vi "Master_IMUMain.vi"(8 "error in":errorcluster, 11 "VISA Refnum out":refnum<visa-resource-name>) -> (0 "error out":errorcluster)   [LabVIEW 2018]
doc: "VI dedicated to reading and processing incoming data from IMU (SBG Ellipse)."
panel:
  out "Data skipped":bool
  out "buffer length":i32
  out "msg_id":string
  # "."
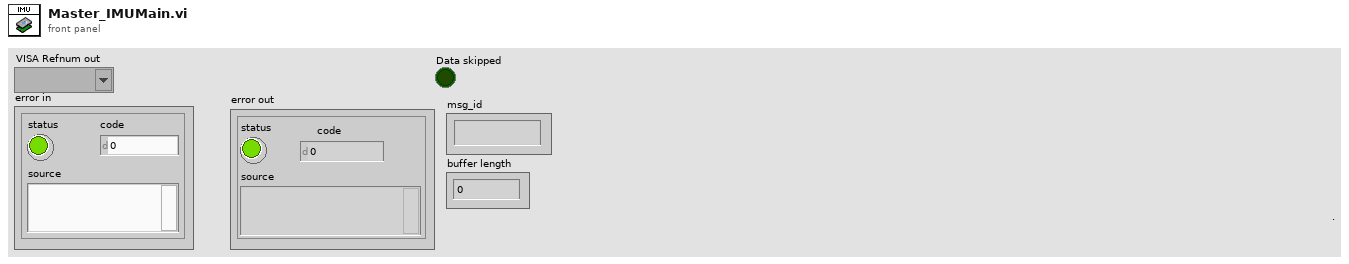
[diagram p1: front panel]
types:
  T1 = cluster{"x acceleration (g)":dbl, "Pressure (psia)":dbl, "Temperature (F)":dbl}
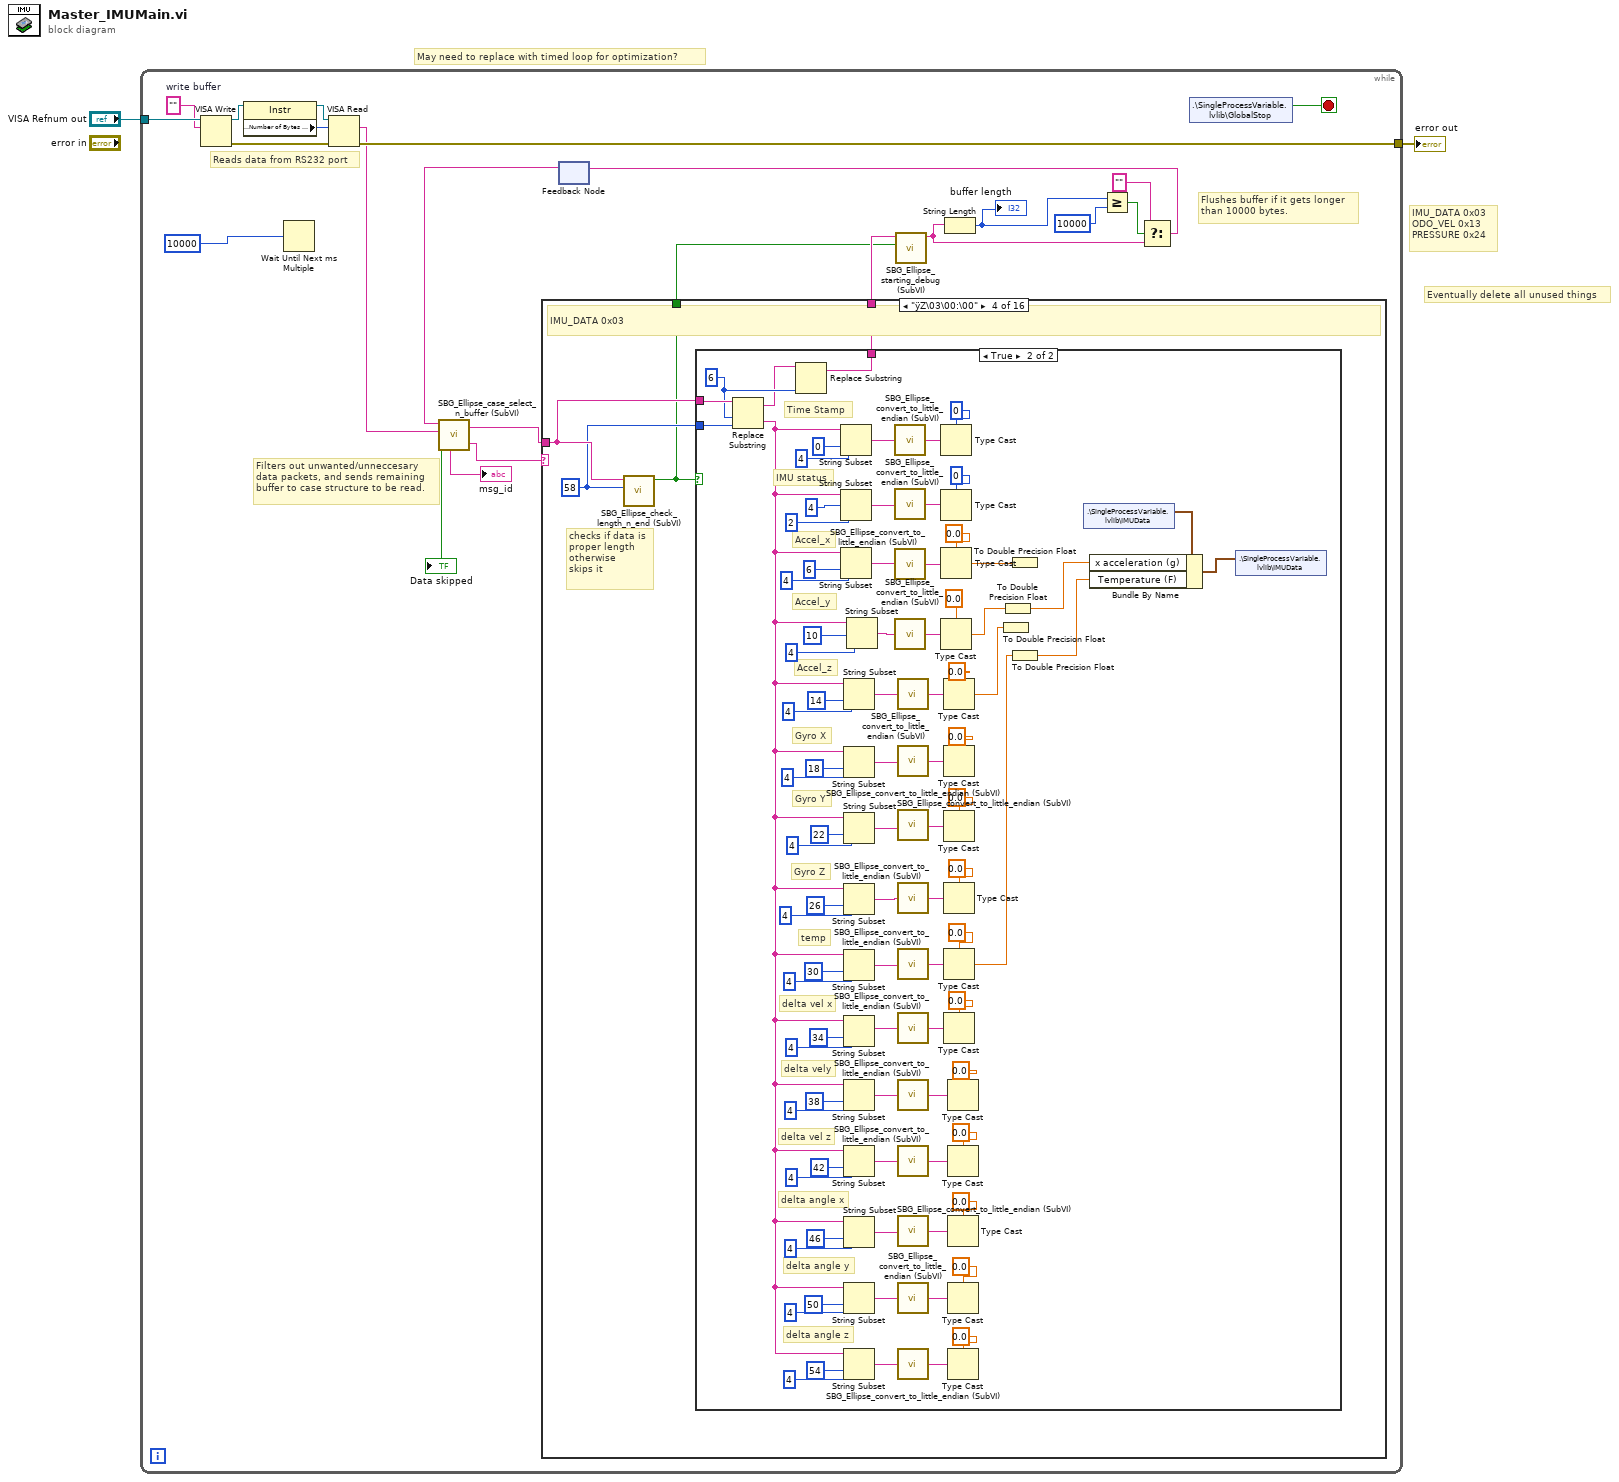
[diagram p0: block diagram]
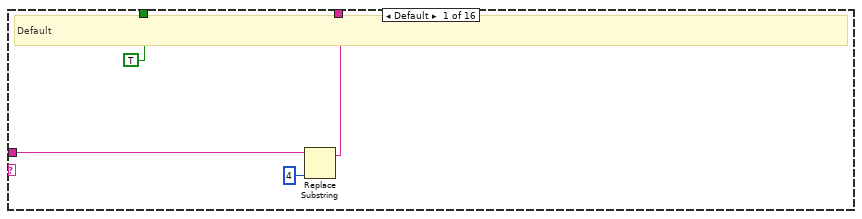
[diagram p2: hidden frame]
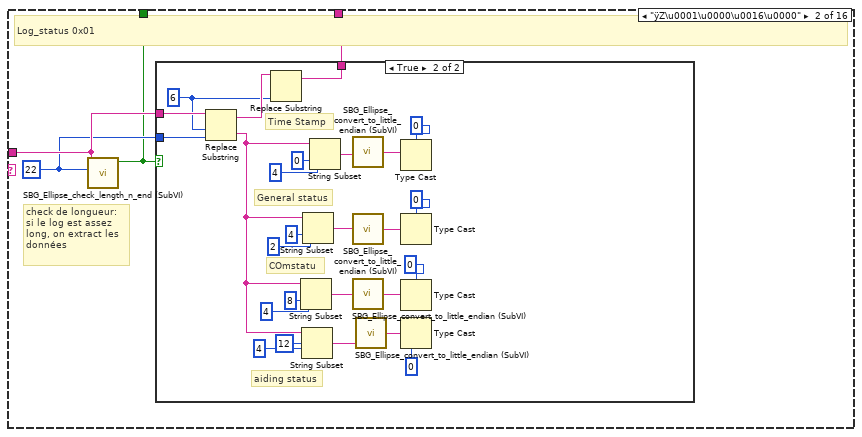
[diagram p3: hidden frame]
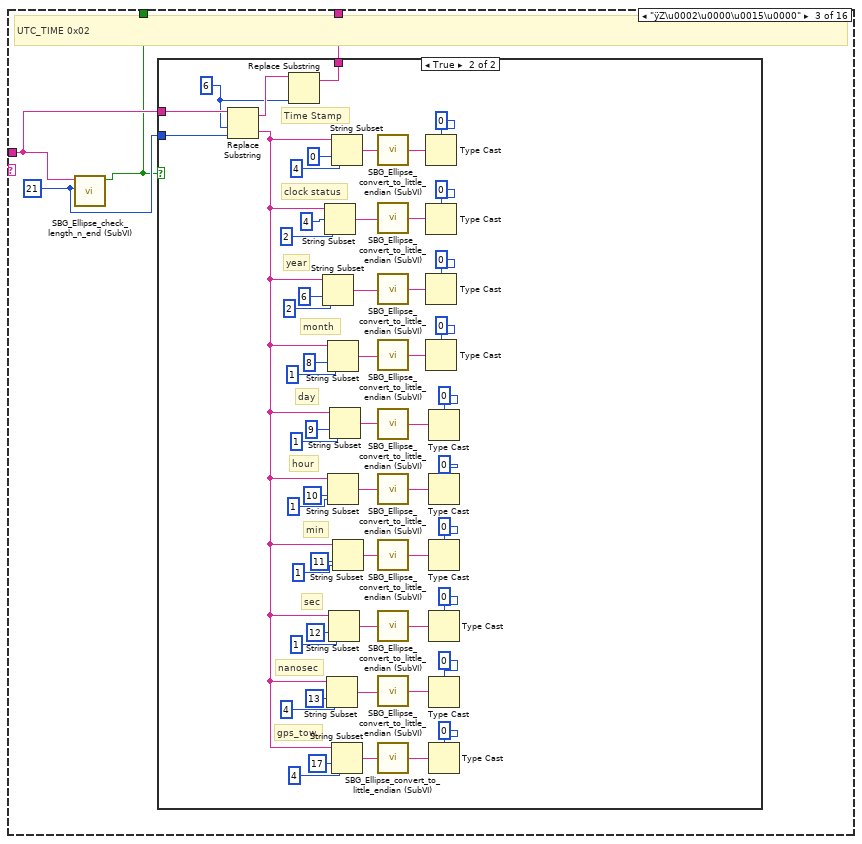
[diagram p5: hidden frame]
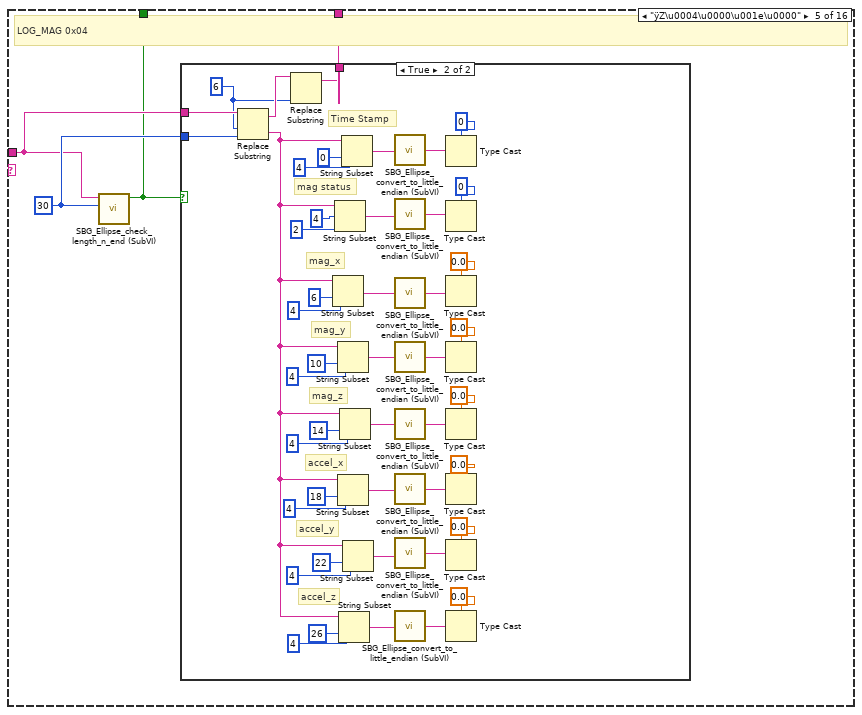
[diagram p8: hidden frame]
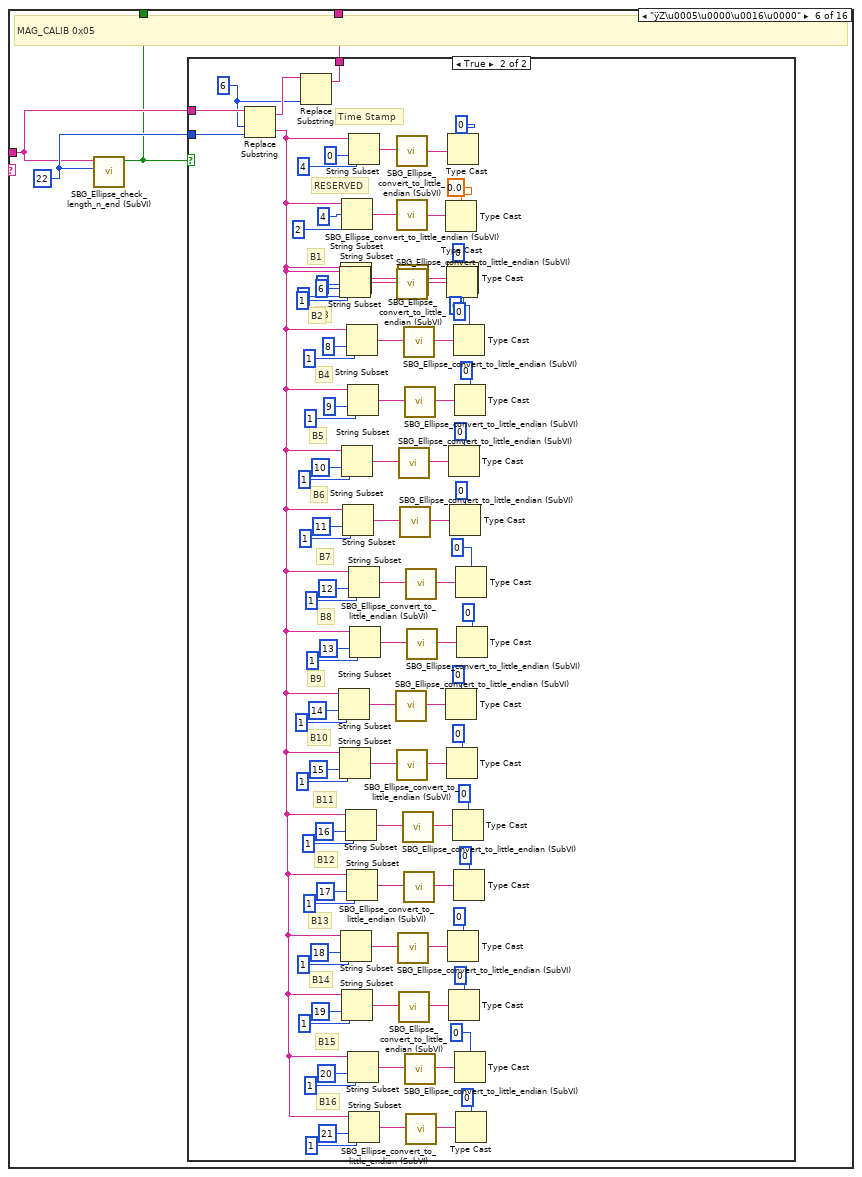
[diagram p10: hidden frame]
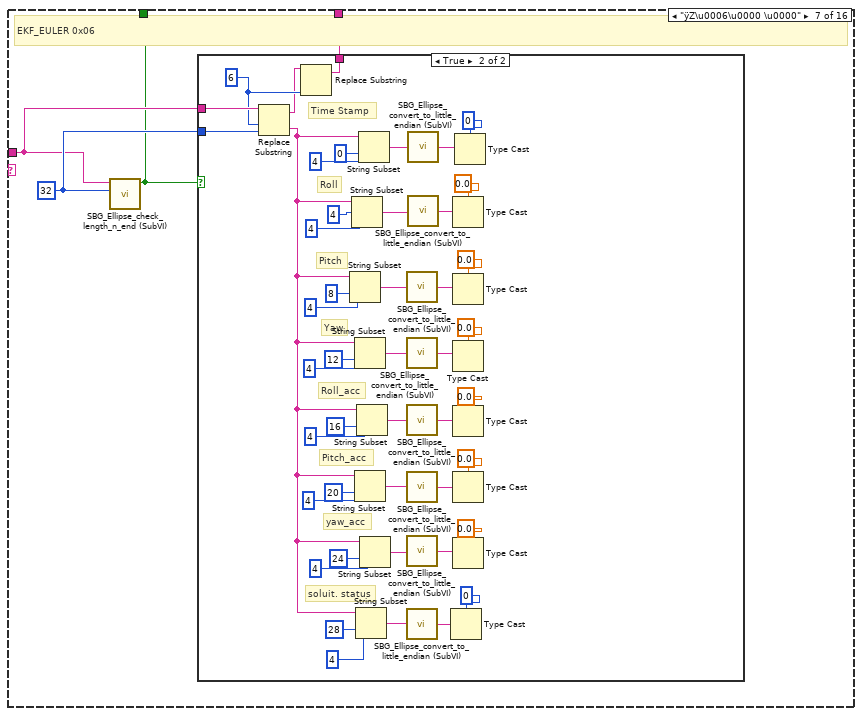
[diagram p12: hidden frame]
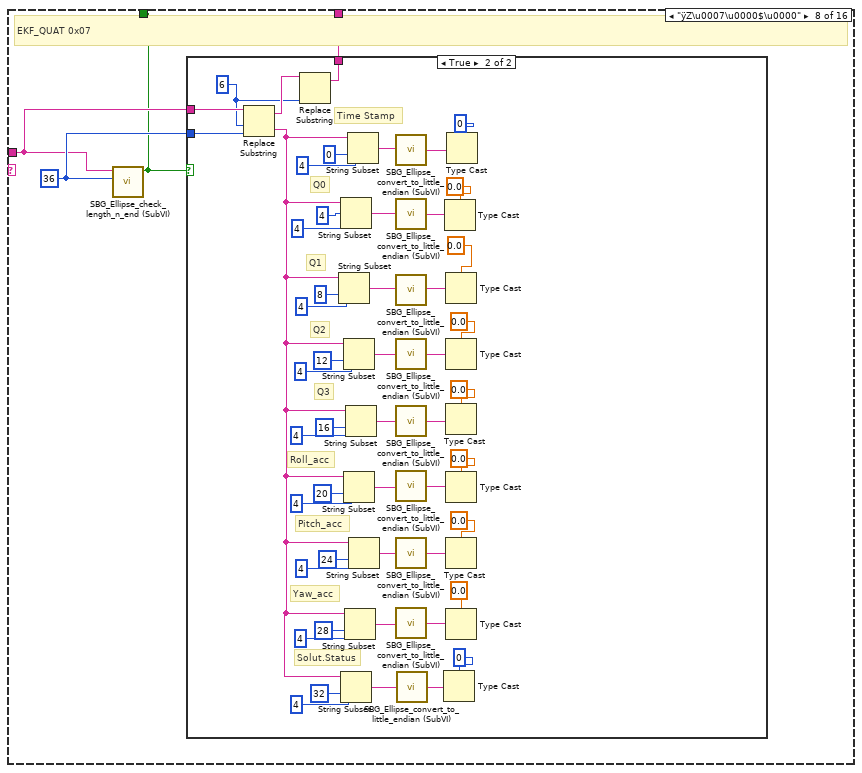
[diagram p14: hidden frame]
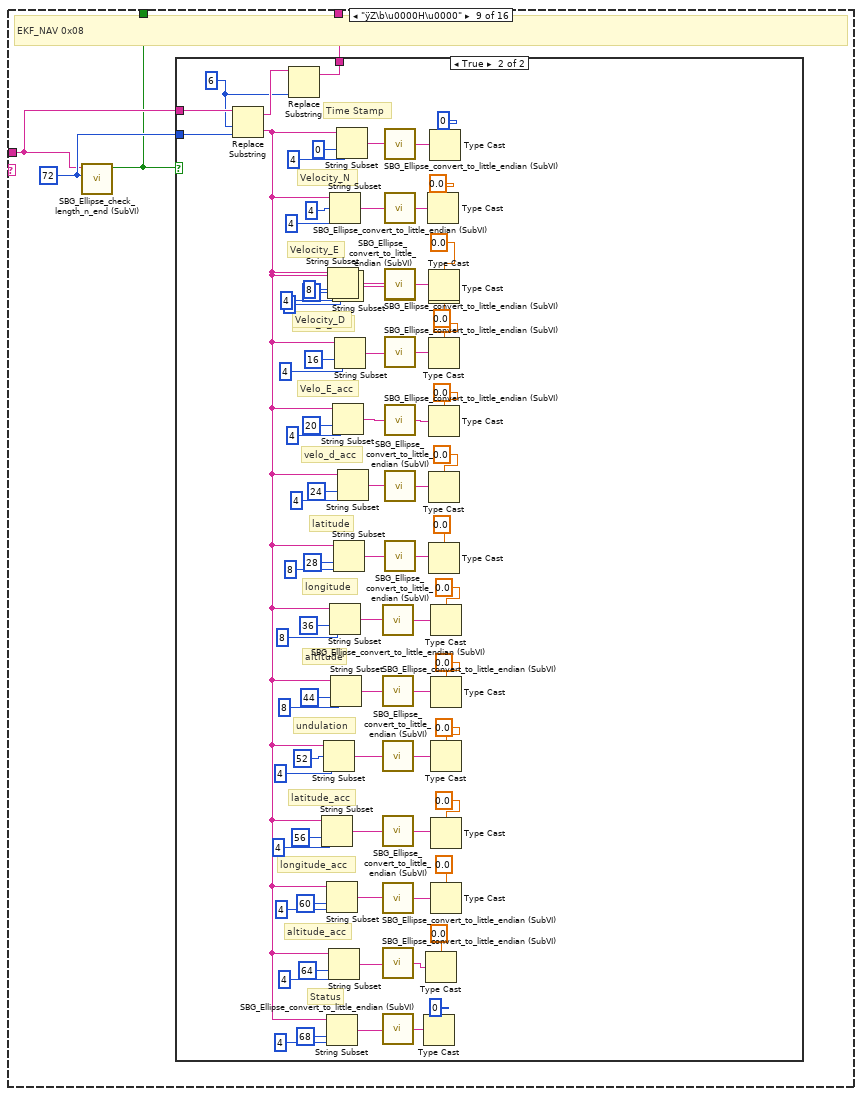
[diagram p16: hidden frame]
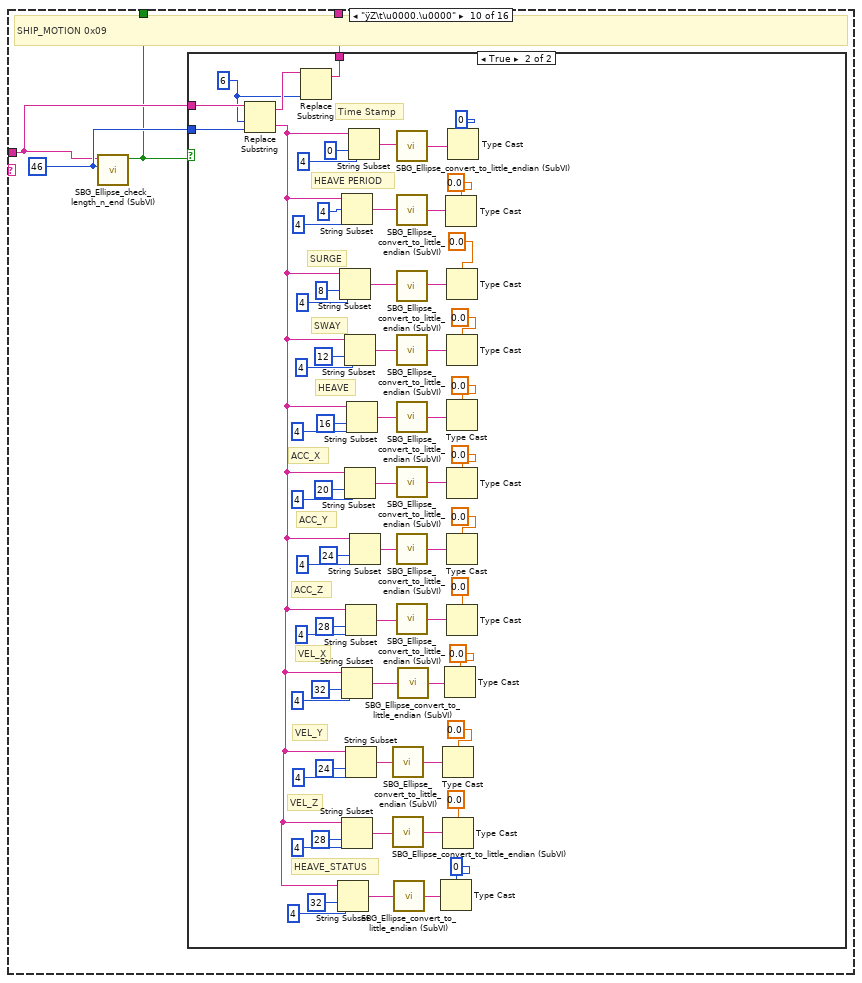
[diagram p18: hidden frame]
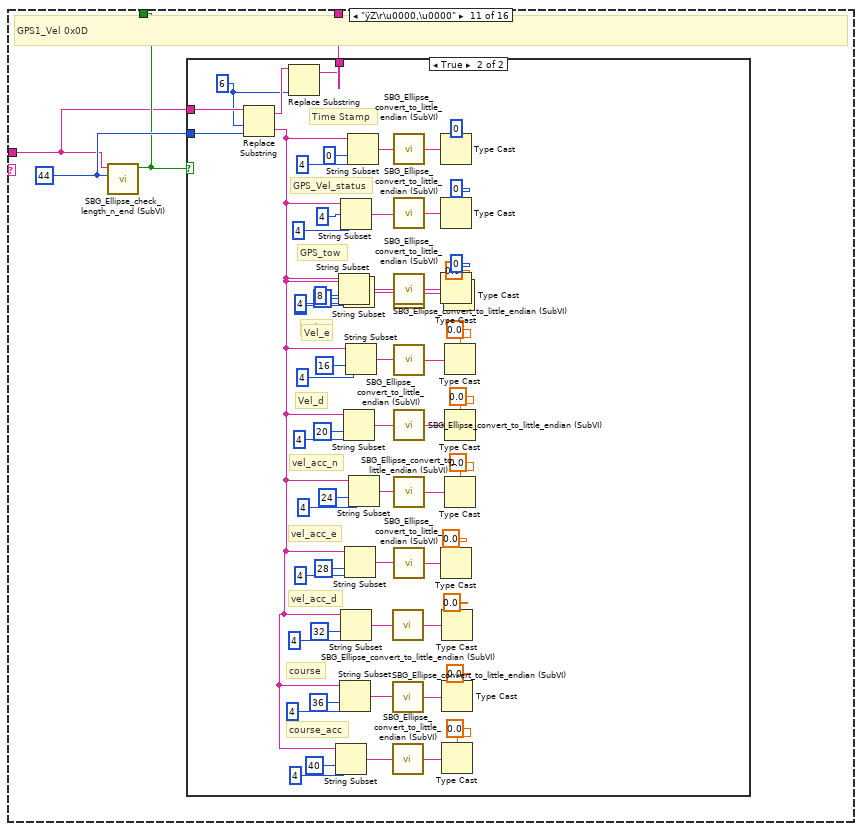
[diagram p20: hidden frame]
diagram:
  # "Eventually delete all unused things"
  # "May need to replace with timed loop for optimization?"
  # "IMU_DATA 0x03\nODO_VEL 0x13\nPRESSURE 0x24"
  n1 = while {
    tunnel: "VISA Refnum out" -> [w25]
    tunnel: [w19] -> w1
    stop <- w9 stop-if-true
    w20 = ""  # write buffer
    # "Filters out unwanted/unneccesary \ndata packets, and sends remaining\nbuffer to case structure to be read."
    # "Reads data from RS232 port"
    # "Flushes buffer if it gets longer\nthan 10000 bytes."
    n2 = VISA Write(VISA resource name=w25, write buffer=w20) -> (VISA resource name out=w21:refnum<visa-resource-name>, error out=w24:errorcluster)  [unwired: 1 in, 1 out]
    n3 = property class="Instr"(reference=w21) -> (reference out=w22:refnum<visa-resource-name>, "Serial Settings:Number of Bytes at Serial Port"=w23:u32)  [unwired: 1 in, 1 out]
    n4 = Wait Until Next ms Multiple(millisecond multiple=u32 10000) -> ()  [unwired: 1 out]
    n5 = VISA Read(VISA resource name=w22, byte count=w23, error in (no error)=w24) -> (read buffer=w17:string, error out=w19:errorcluster)  [unwired: 2 out]
    n6 = feedback #1() -> (w18:string)  [unwired: 1 in]
    n7 = call "SBG_Ellipse_case_select_n_buffer (SubVI).vi"("new data in"=w17, "buffer data in"=w18) -> ("case_selector"=w6:string, "data out"=w7:string, "msg_id"=→"msg_id":string, "Data skipped"=→"Data skipped":bool)  [unwired: 2 in]
    n8 = case shown="\"ÿZ\\03\\00:\\00\"" w6 {
      tunnel: w7 -> [w28 w32 w64 w124 w218 w269 w369 w421 w477 w563 w632 w700 w776 w822 w849 w890]
      tunnel: [w27 w33 w62 w125 w217 w268 w370 w420 w476 w561 w634 w699 w775 w821 w848 w889] -> w8
      tunnel: [TRUE ("Boolean") w30 w61 w122 w216 w267 w368 w419 w475 w562 w633 w698 w774 w820 w847 w888] -> w5
      frame Default {
        # "Default"
        n9 = Replace Substring(2:4 ("length (len. of substring)"), 5:w28) -> (1:w27:string)  [unwired: 2 in, 1 out]
      }
      frame "ÿZ\u0001\u0000\u0016\u0000" {
        w31 = 22 ("x")
        # "check de longueur:\nsi le log est assez\nlong, on extract les \ndonnées"
        # "Log_status 0x01"
        n10 = call "SBG_Ellipse_check_length_n_end (SubVI).vi"("x"=w31, "input String"=w32) -> ("is data ok?"=w30:bool)  [unwired: 7 in, 2 out]
        n11 = case shown="True" w30 {
          tunnel: w32 -> [w34 w60]
          tunnel: [w34 w43] -> w33
          tunnel: w31 -> [_ w50]
          frame False {
          }
          frame True {
            w44 = 6 ("length (len. of substring)")
            # "aiding status"
            # "COmstatu"
            # "General status"
            # "Time Stamp"
            n12 = Replace Substring(2:w50, 3:w44, 5:w60) -> (0:w59:string, 1:w45:string)  [unwired: 1 in]
            n13 = Replace Substring(2:w44, 5:w45) -> (1:w43:string)  [unwired: 2 in, 1 out]
            n14 = String Subset(string=w59, offset (0)=8 ("length (len. of substring)"), length (rest)=4 ("length (len. of substring)")) -> (substring=w41:string)
            n15 = String Subset(string=w59, offset (0)=12 ("length (len. of substring)"), length (rest)=4 ("length (len. of substring)")) -> (substring=w42:string)
            n16 = String Subset(string=w59, offset (0)=4 ("length (len. of substring)"), length (rest)=2 ("length (len. of substring)")) -> (substring=w40:string)
            n17 = String Subset(string=w59, offset (0)=0 ("length (len. of substring)"), length (rest)=4 ("length (len. of substring)")) -> (substring=w39:string)
            n18 = call "SBG_Ellipse_convert_to_little_endian (SubVI).vi"("string"=w39) -> ("String"=w38:string)  [unwired: 4 in]
            n19 = call "SBG_Ellipse_convert_to_little_endian (SubVI).vi"("string"=w40) -> ("String"=w37:string)  [unwired: 4 in]
            n20 = call "SBG_Ellipse_convert_to_little_endian (SubVI).vi"("string"=w41) -> ("String"=w36:string)  [unwired: 4 in]
            n21 = call "SBG_Ellipse_convert_to_little_endian (SubVI).vi"("string"=w42) -> ("String"=w35:string)  [unwired: 4 in]
            n22 = Type Cast(type=u32 0, x=w38) -> ()  [unwired: 1 out]
            n23 = Type Cast(type=u16 0, x=w37) -> ()  [unwired: 1 out]
            n24 = Type Cast(type=u32 0, x=w36) -> ()  [unwired: 1 out]
            n25 = Type Cast(type=u32 0, x=w35) -> ()  [unwired: 1 out]
          }
        }
      }
      frame "ÿZ\u0002\u0000\u0015\u0000" {
        w63 = 21 ("x")
        # "UTC_TIME 0x02"
        n26 = call "SBG_Ellipse_check_length_n_end (SubVI).vi"("x"=w63, "input String"=w64) -> ("is data ok?"=w61:bool)  [unwired: 7 in, 2 out]
        n27 = case shown="True" w61 {
          tunnel: w64 -> [w65 w121]
          tunnel: [w65 w86] -> w62
          tunnel: w63 -> [_ w99]
          frame False {
          }
          frame True {
            w87 = 6 ("length (len. of substring)")
            # "gps_tow"
            # "nanosec"
            # "sec"
            # "min"
            # "hour"
            # "day"
            # "month"
            # "year"
            # "clock status"
            # "Time Stamp"
            n28 = Replace Substring(2:w99, 3:w87, 5:w121) -> (0:w100:string, 1:w88:string)  [unwired: 1 in]
            n29 = Replace Substring(2:w87, 5:w88) -> (1:w86:string)  [unwired: 2 in, 1 out]
            n30 = String Subset(string=w100, offset (0)=6 ("length (len. of substring)"), length (rest)=2 ("length (len. of substring)")) -> (substring=w81:string)
            n31 = String Subset(string=w100, offset (0)=4 ("length (len. of substring)"), length (rest)=2 ("length (len. of substring)")) -> (substring=w83:string)
            n32 = String Subset(string=w100, offset (0)=13 ("length (len. of substring)"), length (rest)=4 ("length (len. of substring)")) -> (substring=w68:string)
            n33 = String Subset(string=w100, offset (0)=8 ("length (len. of substring)"), length (rest)=1 ("length (len. of substring)")) -> (substring=w79:string)
            n34 = String Subset(string=w100, offset (0)=10 ("length (len. of substring)"), length (rest)=1 ("length (len. of substring)")) -> (substring=w75:string)
            n35 = String Subset(string=w100, offset (0)=12 ("length (len. of substring)"), length (rest)=1 ("length (len. of substring)")) -> (substring=w71:string)
            n36 = String Subset(string=w100, offset (0)=9 ("length (len. of substring)"), length (rest)=1 ("length (len. of substring)")) -> (substring=w77:string)
            n37 = String Subset(string=w100, offset (0)=0 ("length (len. of substring)"), length (rest)=4 ("length (len. of substring)")) -> (substring=w85:string)
            n38 = String Subset(string=w100, offset (0)=17 ("length (len. of substring)"), length (rest)=4 ("length (len. of substring)")) -> (substring=w67:string)
            n39 = String Subset(string=w100, offset (0)=11 ("length (len. of substring)"), length (rest)=1 ("length (len. of substring)")) -> (substring=w73:string)
            n40 = call "SBG_Ellipse_convert_to_little_endian (SubVI).vi"("string"=w85) -> ("String"=w84:string)  [unwired: 4 in]
            n41 = call "SBG_Ellipse_convert_to_little_endian (SubVI).vi"("string"=w83) -> ("String"=w82:string)  [unwired: 4 in]
            n42 = call "SBG_Ellipse_convert_to_little_endian (SubVI).vi"("string"=w81) -> ("String"=w80:string)  [unwired: 4 in]
            n43 = call "SBG_Ellipse_convert_to_little_endian (SubVI).vi"("string"=w79) -> ("String"=w78:string)  [unwired: 4 in]
            n44 = call "SBG_Ellipse_convert_to_little_endian (SubVI).vi"("string"=w77) -> ("String"=w76:string)  [unwired: 4 in]
            n45 = call "SBG_Ellipse_convert_to_little_endian (SubVI).vi"("string"=w75) -> ("String"=w74:string)  [unwired: 4 in]
            n46 = call "SBG_Ellipse_convert_to_little_endian (SubVI).vi"("string"=w73) -> ("String"=w72:string)  [unwired: 4 in]
            n47 = call "SBG_Ellipse_convert_to_little_endian (SubVI).vi"("string"=w71) -> ("String"=w70:string)  [unwired: 4 in]
            n48 = call "SBG_Ellipse_convert_to_little_endian (SubVI).vi"("string"=w68) -> ("String"=w69:string)  [unwired: 4 in]
            n49 = call "SBG_Ellipse_convert_to_little_endian (SubVI).vi"("string"=w67) -> ("String"=w66:string)  [unwired: 4 in]
            n50 = Type Cast(type=u32 0, x=w84) -> ()  [unwired: 1 out]
            n51 = Type Cast(type=u16 0, x=w82) -> ()  [unwired: 1 out]
            n52 = Type Cast(type=u16 0, x=w80) -> ()  [unwired: 1 out]
            n53 = Type Cast(type=u8 0, x=w78) -> ()  [unwired: 1 out]
            n54 = Type Cast(type=u8 0, x=w76) -> ()  [unwired: 1 out]
            n55 = Type Cast(type=u8 0, x=w74) -> ()  [unwired: 1 out]
            n56 = Type Cast(type=u8 0, x=w72) -> ()  [unwired: 1 out]
            n57 = Type Cast(type=u8 0, x=w70) -> ()  [unwired: 1 out]
            n58 = Type Cast(type=u32 0, x=w69) -> ()  [unwired: 1 out]
            n59 = Type Cast(type=u32 0, x=w66) -> ()  [unwired: 1 out]
          }
        }
      }
      frame "ÿZ\u0003\u0000:\u0000" {
        w123 = 58 ("x")
        # "checks if data is\nproper length\notherwise\nskips it"
        # "IMU_DATA 0x03"
        n60 = call "SBG_Ellipse_check_length_n_end (SubVI).vi"("x"=w123, "input String"=w124) -> ("is data ok?"=w122:bool)  [unwired: 7 in, 2 out]
        n61 = case shown="True" w122 {
          tunnel: w124 -> [w126 w215]
          tunnel: [w126 w167] -> w125
          tunnel: w123 -> [_ w194]
          frame False {
          }
          frame True {
            w166 = 6 ("length (len. of substring)")
            # "delta angle z"
            # "delta angle y"
            # "delta angle x"
            # "delta vel z"
            # "delta vely"
            # "delta vel x"
            # "temp"
            # "Gyro Z"
            # "Gyro Y"
            # "Gyro X"
            # "Accel_z"
            # "Accel_y"
            # "Accel_x"
            # "IMU status"
            # "Time Stamp"
            n62 = Replace Substring(2:w194, 3:w166, 5:w215) -> (0:w183:string, 1:w165:string)  [unwired: 1 in]
            n63 = Replace Substring(2:w166, 5:w165) -> (1:w167:string)  [unwired: 2 in, 1 out]
            n64 = String Subset(string=w183, offset (0)=0 ("length (len. of substring)"), length (rest)=4 ("length (len. of substring)")) -> (substring=w138:string)
            n65 = String Subset(string=w183, offset (0)=4 ("length (len. of substring)"), length (rest)=2 ("length (len. of substring)")) -> (substring=w137:string)
            n66 = String Subset(string=w183, offset (0)=6 ("length (len. of substring)"), length (rest)=4 ("length (len. of substring)")) -> (substring=w162:string)
            n67 = String Subset(string=w183, offset (0)=14 ("length (len. of substring)"), length (rest)=4 ("length (len. of substring)")) -> (substring=w163:string)
            n68 = String Subset(string=w183, offset (0)=18 ("length (len. of substring)"), length (rest)=4 ("length (len. of substring)")) -> (substring=w143:string)
            n69 = String Subset(string=w183, offset (0)=22 ("length (len. of substring)"), length (rest)=4 ("length (len. of substring)")) -> (substring=w142:string)
            n70 = String Subset(string=w183, offset (0)=26 ("length (len. of substring)"), length (rest)=4 ("length (len. of substring)")) -> (substring=w141:string)
            n71 = String Subset(string=w183, offset (0)=30 ("length (len. of substring)"), length (rest)=4 ("length (len. of substring)")) -> (substring=w146:string)
            n72 = String Subset(string=w183, offset (0)=34 ("length (len. of substring)"), length (rest)=4 ("length (len. of substring)")) -> (substring=w147:string)
            n73 = String Subset(string=w183, offset (0)=38 ("length (len. of substring)"), length (rest)=4 ("length (len. of substring)")) -> (substring=w158:string)
            n74 = String Subset(string=w183, offset (0)=42 ("length (len. of substring)"), length (rest)=4 ("length (len. of substring)")) -> (substring=w151:string)
            n75 = String Subset(string=w183, offset (0)=46 ("length (len. of substring)"), length (rest)=4 ("length (len. of substring)")) -> (substring=w152:string)
            n76 = String Subset(string=w183, offset (0)=50 ("length (len. of substring)"), length (rest)=4 ("length (len. of substring)")) -> (substring=w157:string)
            n77 = String Subset(string=w183, offset (0)=54 ("length (len. of substring)"), length (rest)=4 ("length (len. of substring)")) -> (substring=w156:string)
            n78 = String Subset(string=w183, offset (0)=10 ("length (len. of substring)"), length (rest)=4 ("length (len. of substring)")) -> (substring=w161:string)
            n79 = call "SBG_Ellipse_convert_to_little_endian (SubVI).vi"("string"=w138) -> ("String"=w135:string)  [unwired: 4 in]
            n80 = call "SBG_Ellipse_convert_to_little_endian (SubVI).vi"("string"=w137) -> ("String"=w136:string)  [unwired: 4 in]
            n81 = call "SBG_Ellipse_convert_to_little_endian (SubVI).vi"("string"=w162) -> ("String"=w159:string)  [unwired: 4 in]
            n82 = call "SBG_Ellipse_convert_to_little_endian (SubVI).vi"("string"=w161) -> ("String"=w160:string)  [unwired: 4 in]
            n83 = call "SBG_Ellipse_convert_to_little_endian (SubVI).vi"("string"=w163) -> ("String"=w164:string)  [unwired: 4 in]
            n84 = call "SBG_Ellipse_convert_to_little_endian (SubVI).vi"("string"=w143) -> ("String"=w144:string)  [unwired: 4 in]
            n85 = call "SBG_Ellipse_convert_to_little_endian (SubVI).vi"("string"=w142) -> ("String"=w139:string)  [unwired: 4 in]
            n86 = call "SBG_Ellipse_convert_to_little_endian (SubVI).vi"("string"=w141) -> ("String"=w140:string)  [unwired: 4 in]
            n87 = call "SBG_Ellipse_convert_to_little_endian (SubVI).vi"("string"=w146) -> ("String"=w145:string)  [unwired: 4 in]
            n88 = call "SBG_Ellipse_convert_to_little_endian (SubVI).vi"("string"=w147) -> ("String"=w148:string)  [unwired: 4 in]
            n89 = call "SBG_Ellipse_convert_to_little_endian (SubVI).vi"("string"=w158) -> ("String"=w149:string)  [unwired: 4 in]
            n90 = call "SBG_Ellipse_convert_to_little_endian (SubVI).vi"("string"=w151) -> ("String"=w150:string)  [unwired: 4 in]
            n91 = call "SBG_Ellipse_convert_to_little_endian (SubVI).vi"("string"=w152) -> ("String"=w153:string)  [unwired: 4 in]
            n92 = call "SBG_Ellipse_convert_to_little_endian (SubVI).vi"("string"=w157) -> ("String"=w154:string)  [unwired: 4 in]
            n93 = call "SBG_Ellipse_convert_to_little_endian (SubVI).vi"("string"=w156) -> ("String"=w155:string)  [unwired: 4 in]
            n94 = Type Cast(type=u32 0, x=w135) -> ()  [unwired: 1 out]
            n95 = Type Cast(type=u16 0, x=w136) -> ()  [unwired: 1 out]
            n96 = Type Cast(type=sgl 0.0, x=w159) -> (*(type *) &x=w134:sgl)
            n97 = Type Cast(type=sgl 0.0, x=w160) -> (*(type *) &x=w130:sgl)
            n98 = Type Cast(type=sgl 0.0, x=w164) -> (*(type *) &x=w129:sgl)
            n99 = Type Cast(type=sgl 0.0, x=w144) -> ()  [unwired: 1 out]
            n100 = Type Cast(type=sgl 0.0, x=w139) -> ()  [unwired: 1 out]
            n101 = Type Cast(type=sgl 0.0, x=w140) -> ()  [unwired: 1 out]
            n102 = Type Cast(type=sgl 0.0, x=w145) -> (*(type *) &x=w133:sgl)
            n103 = Type Cast(type=sgl 0.0, x=w148) -> ()  [unwired: 1 out]
            n104 = Type Cast(type=sgl 0.0, x=w149) -> ()  [unwired: 1 out]
            n105 = Type Cast(type=sgl 0.0, x=w150) -> ()  [unwired: 1 out]
            n106 = Type Cast(type=sgl 0.0, x=w153) -> ()  [unwired: 1 out]
            n107 = Type Cast(type=sgl 0.0, x=w154) -> ()  [unwired: 1 out]
            n108 = Type Cast(type=sgl 0.0, x=w155) -> ()  [unwired: 1 out]
            n109 = To Double Precision Float(number=w129) -> ()  [unwired: 1 out]
            n110 = To Double Precision Float(number=w130) -> (double precision float=w128:dbl)
            n111 = To Double Precision Float(number=w134) -> ()  [unwired: 1 out]
            n112 = To Double Precision Float(number=w133) -> (double precision float=w131:dbl)
            n113 = shared-variable ".\\SingleProcessVariable.lvlib\\IMUData"() -> (w127:T1)  [unwired: 1 in, 1 out]
            n114 = Bundle By Name(cluster=w127, "x acceleration (g)"=w128, "Temperature (F)"=w131) -> (w132:T1)
            n115 = shared-variable ".\\SingleProcessVariable.lvlib\\IMUData"(w132) -> ()  [unwired: 1 in, 1 out]
          }
        }
      }
      frame "ÿZ\u0004\u0000\u001e\u0000" {
        w219 = 30 ("x")
        # "LOG_MAG 0x04"
        n116 = call "SBG_Ellipse_check_length_n_end (SubVI).vi"("x"=w219, "input String"=w218) -> ("is data ok?"=w216:bool)  [unwired: 7 in, 2 out]
        n117 = case shown="True" w216 {
          tunnel: w218 -> [w220 w266]
          tunnel: [w220 w237] -> w217
          tunnel: w219 -> [_ w248]
          frame False {
          }
          frame True {
            w238 = 6 ("length (len. of substring)")
            # "accel_z"
            # "accel_y"
            # "accel_x"
            # "mag_z"
            # "mag_y"
            # "mag_x"
            # "mag status"
            # "Time Stamp"
            n118 = Replace Substring(2:w248, 3:w238, 5:w266) -> (0:w249:string, 1:w239:string)  [unwired: 1 in]
            n119 = Replace Substring(2:w238, 5:w239) -> (1:w237:string)  [unwired: 2 in, 1 out]
            n120 = String Subset(string=w249, offset (0)=6 ("length (len. of substring)"), length (rest)=4 ("length (len. of substring)")) -> (substring=w232:string)
            n121 = String Subset(string=w249, offset (0)=4 ("length (len. of substring)"), length (rest)=2 ("length (len. of substring)")) -> (substring=w234:string)
            n122 = String Subset(string=w249, offset (0)=10 ("length (len. of substring)"), length (rest)=4 ("length (len. of substring)")) -> (substring=w229:string)
            n123 = String Subset(string=w249, offset (0)=18 ("length (len. of substring)"), length (rest)=4 ("length (len. of substring)")) -> (substring=w226:string)
            n124 = String Subset(string=w249, offset (0)=26 ("length (len. of substring)"), length (rest)=4 ("length (len. of substring)")) -> (substring=w224:string)
            n125 = String Subset(string=w249, offset (0)=14 ("length (len. of substring)"), length (rest)=4 ("length (len. of substring)")) -> (substring=w228:string)
            n126 = String Subset(string=w249, offset (0)=0 ("length (len. of substring)"), length (rest)=4 ("length (len. of substring)")) -> (substring=w236:string)
            n127 = String Subset(string=w249, offset (0)=22 ("length (len. of substring)"), length (rest)=4 ("length (len. of substring)")) -> (substring=w225:string)
            n128 = call "SBG_Ellipse_convert_to_little_endian (SubVI).vi"("string"=w236) -> ("String"=w235:string)  [unwired: 4 in]
            n129 = call "SBG_Ellipse_convert_to_little_endian (SubVI).vi"("string"=w234) -> ("String"=w233:string)  [unwired: 4 in]
            n130 = call "SBG_Ellipse_convert_to_little_endian (SubVI).vi"("string"=w232) -> ("String"=w231:string)  [unwired: 4 in]
            n131 = call "SBG_Ellipse_convert_to_little_endian (SubVI).vi"("string"=w229) -> ("String"=w230:string)  [unwired: 4 in]
            n132 = call "SBG_Ellipse_convert_to_little_endian (SubVI).vi"("string"=w228) -> ("String"=w227:string)  [unwired: 4 in]
            n133 = call "SBG_Ellipse_convert_to_little_endian (SubVI).vi"("string"=w226) -> ("String"=w221:string)  [unwired: 4 in]
            n134 = call "SBG_Ellipse_convert_to_little_endian (SubVI).vi"("string"=w225) -> ("String"=w222:string)  [unwired: 4 in]
            n135 = call "SBG_Ellipse_convert_to_little_endian (SubVI).vi"("string"=w224) -> ("String"=w223:string)  [unwired: 4 in]
            n136 = Type Cast(type=u32 0, x=w235) -> ()  [unwired: 1 out]
            n137 = Type Cast(type=u16 0, x=w233) -> ()  [unwired: 1 out]
            n138 = Type Cast(type=sgl 0.0, x=w231) -> ()  [unwired: 1 out]
            n139 = Type Cast(type=sgl 0.0, x=w230) -> ()  [unwired: 1 out]
            n140 = Type Cast(type=sgl 0.0, x=w227) -> ()  [unwired: 1 out]
            n141 = Type Cast(type=sgl 0.0, x=w221) -> ()  [unwired: 1 out]
            n142 = Type Cast(type=sgl 0.0, x=w222) -> ()  [unwired: 1 out]
            n143 = Type Cast(type=sgl 0.0, x=w223) -> ()  [unwired: 1 out]
          }
        }
      }
      frame "ÿZ\u0005\u0000\u0016\u0000" {
        w270 = 22 ("x")
        # "MAG_CALIB 0x05"
        n144 = call "SBG_Ellipse_check_length_n_end (SubVI).vi"("x"=w270, "input String"=w269) -> ("is data ok?"=w267:bool)  [unwired: 7 in, 2 out]
        n145 = case shown="True" w267 {
          tunnel: w269 -> [w271 w367]
          tunnel: [w271 w354] -> w268
          tunnel: w270 -> [_ w360]
          frame False {
          }
          frame True {
            w355 = 6 ("length (len. of substring)")
            # "B16"
            # "B15"
            # "B14"
            # "B13"
            # "B12"
            # "B11"
            # "B10"
            # "B9"
            # "B8"
            # "B7"
            # "B6"
            # "B5"
            # "B4"
            # "B3"
            # "B2"
            # "B1"
            # "RESERVED"
            # "Time Stamp"
            n146 = Replace Substring(2:w360, 3:w355, 5:w367) -> (0:w272:string, 1:w356:string)  [unwired: 1 in]
            n147 = Replace Substring(2:w355, 5:w356) -> (1:w354:string)  [unwired: 2 in, 1 out]
            n148 = String Subset(string=w272, offset (0)=14 ("length (len. of substring)"), length (rest)=1 ("length (len. of substring)")) -> (substring=w276:string)
            n149 = String Subset(string=w272, offset (0)=6 ("length (len. of substring)"), length (rest)=1 ("length (len. of substring)")) -> (substring=w349:string)
            n150 = String Subset(string=w272, offset (0)=15 ("length (len. of substring)"), length (rest)=1 ("length (len. of substring)")) -> (substring=w279:string)
            n151 = String Subset(string=w272, offset (0)=7 ("length (len. of substring)"), length (rest)=1 ("length (len. of substring)")) -> (substring=w346:string)
            n152 = String Subset(string=w272, offset (0)=18 ("length (len. of substring)"), length (rest)=1 ("length (len. of substring)")) -> (substring=w309:string)
            n153 = String Subset(string=w272, offset (0)=4 ("length (len. of substring)"), length (rest)=2 ("length (len. of substring)")) -> (substring=w351:string)
            n154 = String Subset(string=w272, offset (0)=10 ("length (len. of substring)"), length (rest)=1 ("length (len. of substring)")) -> (substring=w316:string)
            n155 = String Subset(string=w272, offset (0)=19 ("length (len. of substring)"), length (rest)=1 ("length (len. of substring)")) -> (substring=w306:string)
            n156 = String Subset(string=w272, offset (0)=11 ("length (len. of substring)"), length (rest)=1 ("length (len. of substring)")) -> (substring=w319:string)
            n157 = String Subset(string=w272, offset (0)=16 ("length (len. of substring)"), length (rest)=1 ("length (len. of substring)")) -> (substring=w287:string)
            n158 = String Subset(string=w272, offset (0)=8 ("length (len. of substring)"), length (rest)=1 ("length (len. of substring)")) -> (substring=w338:string)
            n159 = String Subset(string=w272, offset (0)=17 ("length (len. of substring)"), length (rest)=1 ("length (len. of substring)")) -> (substring=w284:string)
            n160 = String Subset(string=w272, offset (0)=9 ("length (len. of substring)"), length (rest)=1 ("length (len. of substring)")) -> (substring=w341:string)
            n161 = String Subset(string=w272, offset (0)=20 ("length (len. of substring)"), length (rest)=1 ("length (len. of substring)")) -> (substring=w298:string)
            n162 = String Subset(string=w272, offset (0)=0 ("length (len. of substring)"), length (rest)=4 ("length (len. of substring)")) -> (substring=w353:string)
            n163 = String Subset(string=w272, offset (0)=12 ("length (len. of substring)"), length (rest)=1 ("length (len. of substring)")) -> (substring=w327:string)
            n164 = String Subset(string=w272, offset (0)=21 ("length (len. of substring)"), length (rest)=1 ("length (len. of substring)")) -> (substring=w301:string)
            n165 = String Subset(string=w272, offset (0)=13 ("length (len. of substring)"), length (rest)=1 ("length (len. of substring)")) -> (substring=w324:string)
            n166 = call "SBG_Ellipse_convert_to_little_endian (SubVI).vi"("string"=w276) -> ("String"=w277:string)  [unwired: 4 in]
            n167 = call "SBG_Ellipse_convert_to_little_endian (SubVI).vi"("string"=w353) -> ("String"=w352:string)  [unwired: 4 in]
            n168 = call "SBG_Ellipse_convert_to_little_endian (SubVI).vi"("string"=w351) -> ("String"=w350:string)  [unwired: 4 in]
            n169 = call "SBG_Ellipse_convert_to_little_endian (SubVI).vi"("string"=w349) -> ("String"=w348:string)  [unwired: 4 in]
            n170 = call "SBG_Ellipse_convert_to_little_endian (SubVI).vi"("string"=w279) -> ("String"=w278:string)  [unwired: 4 in]
            n171 = call "SBG_Ellipse_convert_to_little_endian (SubVI).vi"("string"=w346) -> ("String"=w347:string)  [unwired: 4 in]
            n172 = call "SBG_Ellipse_convert_to_little_endian (SubVI).vi"("string"=w309) -> ("String"=w308:string)  [unwired: 4 in]
            n173 = call "SBG_Ellipse_convert_to_little_endian (SubVI).vi"("string"=w316) -> ("String"=w317:string)  [unwired: 4 in]
            n174 = call "SBG_Ellipse_convert_to_little_endian (SubVI).vi"("string"=w306) -> ("String"=w307:string)  [unwired: 4 in]
            n175 = call "SBG_Ellipse_convert_to_little_endian (SubVI).vi"("string"=w319) -> ("String"=w318:string)  [unwired: 4 in]
            n176 = call "SBG_Ellipse_convert_to_little_endian (SubVI).vi"("string"=w287) -> ("String"=w286:string)  [unwired: 4 in]
            n177 = call "SBG_Ellipse_convert_to_little_endian (SubVI).vi"("string"=w338) -> ("String"=w339:string)  [unwired: 4 in]
            n178 = call "SBG_Ellipse_convert_to_little_endian (SubVI).vi"("string"=w284) -> ("String"=w285:string)  [unwired: 4 in]
            n179 = call "SBG_Ellipse_convert_to_little_endian (SubVI).vi"("string"=w341) -> ("String"=w340:string)  [unwired: 4 in]
            n180 = call "SBG_Ellipse_convert_to_little_endian (SubVI).vi"("string"=w298) -> ("String"=w299:string)  [unwired: 4 in]
            n181 = call "SBG_Ellipse_convert_to_little_endian (SubVI).vi"("string"=w327) -> ("String"=w326:string)  [unwired: 4 in]
            n182 = call "SBG_Ellipse_convert_to_little_endian (SubVI).vi"("string"=w301) -> ("String"=w300:string)  [unwired: 4 in]
            n183 = call "SBG_Ellipse_convert_to_little_endian (SubVI).vi"("string"=w324) -> ("String"=w325:string)  [unwired: 4 in]
            n184 = Type Cast(type=sgl 0.0, x=w350) -> ()  [unwired: 1 out]
            n185 = Type Cast(type=u8 0, x=w277) -> ()  [unwired: 1 out]
            n186 = Type Cast(type=u8 0, x=w348) -> ()  [unwired: 1 out]
            n187 = Type Cast(type=u8 0, x=w278) -> ()  [unwired: 1 out]
            n188 = Type Cast(type=u32 0, x=w352) -> ()  [unwired: 1 out]
            n189 = Type Cast(type=u8 0, x=w347) -> ()  [unwired: 1 out]
            n190 = Type Cast(type=u8 0, x=w308) -> ()  [unwired: 1 out]
            n191 = Type Cast(type=u8 0, x=w317) -> ()  [unwired: 1 out]
            n192 = Type Cast(type=u8 0, x=w307) -> ()  [unwired: 1 out]
            n193 = Type Cast(type=u8 0, x=w318) -> ()  [unwired: 1 out]
            n194 = Type Cast(type=u8 0, x=w286) -> ()  [unwired: 1 out]
            n195 = Type Cast(type=u8 0, x=w339) -> ()  [unwired: 1 out]
            n196 = Type Cast(type=u8 0, x=w285) -> ()  [unwired: 1 out]
            n197 = Type Cast(type=u8 0, x=w340) -> ()  [unwired: 1 out]
            n198 = Type Cast(type=u8 0, x=w299) -> ()  [unwired: 1 out]
            n199 = Type Cast(type=u8 0, x=w326) -> ()  [unwired: 1 out]
            n200 = Type Cast(type=u8 0, x=w300) -> ()  [unwired: 1 out]
            n201 = Type Cast(type=u8 0, x=w325) -> ()  [unwired: 1 out]
          }
        }
      }
      frame "ÿZ\u0006\u0000 \u0000" {
        w371 = 32 ("x")
        # "EKF_EULER 0x06"
        n202 = call "SBG_Ellipse_check_length_n_end (SubVI).vi"("x"=w371, "input String"=w369) -> ("is data ok?"=w368:bool)  [unwired: 7 in, 2 out]
        n203 = case shown="True" w368 {
          tunnel: w369 -> [w372 w418]
          tunnel: [w372 w390] -> w370
          tunnel: w371 -> [_ w400]
          frame False {
          }
          frame True {
            w391 = 6 ("length (len. of substring)")
            # "soluit. status"
            # "yaw_acc"
            # "Pitch_acc"
            # "Roll_acc"
            # "Yaw"
            # "Pitch"
            # "Roll"
            # "Time Stamp"
            n204 = Replace Substring(2:w400, 3:w391, 5:w418) -> (0:w401:string, 1:w389:string)  [unwired: 1 in]
            n205 = Replace Substring(2:w391, 5:w389) -> (1:w390:string)  [unwired: 2 in, 1 out]
            n206 = String Subset(string=w401, offset (0)=8 ("length (len. of substring)"), length (rest)=4 ("length (len. of substring)")) -> (substring=w384:string)
            n207 = String Subset(string=w401, offset (0)=4 ("length (len. of substring)"), length (rest)=4 ("length (len. of substring)")) -> (substring=w386:string)
            n208 = String Subset(string=w401, offset (0)=12 ("length (len. of substring)"), length (rest)=4 ("length (len. of substring)")) -> (substring=w382:string)
            n209 = String Subset(string=w401, offset (0)=20 ("length (len. of substring)"), length (rest)=4 ("length (len. of substring)")) -> (substring=w378:string)
            n210 = String Subset(string=w401, offset (0)=28 ("length (len. of substring)"), length (rest)=4 ("length (len. of substring)")) -> (substring=w374:string)
            n211 = String Subset(string=w401, offset (0)=16 ("length (len. of substring)"), length (rest)=4 ("length (len. of substring)")) -> (substring=w380:string)
            n212 = String Subset(string=w401, offset (0)=0 ("length (len. of substring)"), length (rest)=4 ("length (len. of substring)")) -> (substring=w388:string)
            n213 = String Subset(string=w401, offset (0)=24 ("length (len. of substring)"), length (rest)=4 ("length (len. of substring)")) -> (substring=w376:string)
            n214 = call "SBG_Ellipse_convert_to_little_endian (SubVI).vi"("string"=w384) -> ("String"=w383:string)  [unwired: 4 in]
            n215 = call "SBG_Ellipse_convert_to_little_endian (SubVI).vi"("string"=w382) -> ("String"=w381:string)  [unwired: 4 in]
            n216 = call "SBG_Ellipse_convert_to_little_endian (SubVI).vi"("string"=w380) -> ("String"=w379:string)  [unwired: 4 in]
            n217 = call "SBG_Ellipse_convert_to_little_endian (SubVI).vi"("string"=w378) -> ("String"=w377:string)  [unwired: 4 in]
            n218 = call "SBG_Ellipse_convert_to_little_endian (SubVI).vi"("string"=w376) -> ("String"=w375:string)  [unwired: 4 in]
            n219 = call "SBG_Ellipse_convert_to_little_endian (SubVI).vi"("string"=w374) -> ("String"=w373:string)  [unwired: 4 in]
            n220 = call "SBG_Ellipse_convert_to_little_endian (SubVI).vi"("string"=w388) -> ("String"=w387:string)  [unwired: 4 in]
            n221 = call "SBG_Ellipse_convert_to_little_endian (SubVI).vi"("string"=w386) -> ("String"=w385:string)  [unwired: 4 in]
            n222 = Type Cast(type=u32 0, x=w373) -> ()  [unwired: 1 out]
            n223 = Type Cast(type=sgl 0.0, x=w385) -> ()  [unwired: 1 out]
            n224 = Type Cast(type=sgl 0.0, x=w383) -> ()  [unwired: 1 out]
            n225 = Type Cast(type=sgl 0.0, x=w381) -> ()  [unwired: 1 out]
            n226 = Type Cast(type=sgl 0.0, x=w379) -> ()  [unwired: 1 out]
            n227 = Type Cast(type=sgl 0.0, x=w377) -> ()  [unwired: 1 out]
            n228 = Type Cast(type=sgl 0.0, x=w375) -> ()  [unwired: 1 out]
            n229 = Type Cast(type=u32 0, x=w387) -> ()  [unwired: 1 out]
          }
        }
      }
      frame "ÿZ\u0007\u0000$\u0000" {
        w422 = 36 ("x")
        # "EKF_QUAT 0x07"
        n230 = call "SBG_Ellipse_check_length_n_end (SubVI).vi"("x"=w422, "input String"=w421) -> ("is data ok?"=w419:bool)  [unwired: 7 in, 2 out]
        n231 = case shown="True" w419 {
          tunnel: w421 -> [w423 w474]
          tunnel: [w423 w442] -> w420
          tunnel: w422 -> [_ w457]
          frame False {
          }
          frame True {
            w443 = 6 ("length (len. of substring)")
            # "Solut.Status"
            # "Yaw_acc"
            # "Pitch_acc"
            # "Roll_acc"
            # "Q3"
            # "Q2"
            # "Q1"
            # "Q0"
            # "Time Stamp"
            n232 = Replace Substring(2:w457, 3:w443, 5:w474) -> (0:w454:string, 1:w444:string)  [unwired: 1 in]
            n233 = Replace Substring(2:w443, 5:w444) -> (1:w442:string)  [unwired: 2 in, 1 out]
            n234 = String Subset(string=w454, offset (0)=8 ("length (len. of substring)"), length (rest)=4 ("length (len. of substring)")) -> (substring=w437:string)
            n235 = String Subset(string=w454, offset (0)=4 ("length (len. of substring)"), length (rest)=4 ("length (len. of substring)")) -> (substring=w439:string)
            n236 = String Subset(string=w454, offset (0)=32 ("length (len. of substring)"), length (rest)=4 ("length (len. of substring)")) -> (substring=w424:string)
            n237 = String Subset(string=w454, offset (0)=12 ("length (len. of substring)"), length (rest)=4 ("length (len. of substring)")) -> (substring=w435:string)
            n238 = String Subset(string=w454, offset (0)=20 ("length (len. of substring)"), length (rest)=4 ("length (len. of substring)")) -> (substring=w431:string)
            n239 = String Subset(string=w454, offset (0)=28 ("length (len. of substring)"), length (rest)=4 ("length (len. of substring)")) -> (substring=w427:string)
            n240 = String Subset(string=w454, offset (0)=16 ("length (len. of substring)"), length (rest)=4 ("length (len. of substring)")) -> (substring=w433:string)
            n241 = String Subset(string=w454, offset (0)=0 ("length (len. of substring)"), length (rest)=4 ("length (len. of substring)")) -> (substring=w441:string)
            n242 = String Subset(string=w454, offset (0)=24 ("length (len. of substring)"), length (rest)=4 ("length (len. of substring)")) -> (substring=w429:string)
            n243 = call "SBG_Ellipse_convert_to_little_endian (SubVI).vi"("string"=w441) -> ("String"=w440:string)  [unwired: 4 in]
            n244 = call "SBG_Ellipse_convert_to_little_endian (SubVI).vi"("string"=w439) -> ("String"=w438:string)  [unwired: 4 in]
            n245 = call "SBG_Ellipse_convert_to_little_endian (SubVI).vi"("string"=w437) -> ("String"=w436:string)  [unwired: 4 in]
            n246 = call "SBG_Ellipse_convert_to_little_endian (SubVI).vi"("string"=w435) -> ("String"=w434:string)  [unwired: 4 in]
            n247 = call "SBG_Ellipse_convert_to_little_endian (SubVI).vi"("string"=w433) -> ("String"=w432:string)  [unwired: 4 in]
            n248 = call "SBG_Ellipse_convert_to_little_endian (SubVI).vi"("string"=w431) -> ("String"=w430:string)  [unwired: 4 in]
            n249 = call "SBG_Ellipse_convert_to_little_endian (SubVI).vi"("string"=w429) -> ("String"=w428:string)  [unwired: 4 in]
            n250 = call "SBG_Ellipse_convert_to_little_endian (SubVI).vi"("string"=w427) -> ("String"=w426:string)  [unwired: 4 in]
            n251 = call "SBG_Ellipse_convert_to_little_endian (SubVI).vi"("string"=w424) -> ("String"=w425:string)  [unwired: 4 in]
            n252 = Type Cast(type=u32 0, x=w425) -> ()  [unwired: 1 out]
            n253 = Type Cast(type=sgl 0.0, x=w438) -> ()  [unwired: 1 out]
            n254 = Type Cast(type=sgl 0.0, x=w436) -> ()  [unwired: 1 out]
            n255 = Type Cast(type=sgl 0.0, x=w434) -> ()  [unwired: 1 out]
            n256 = Type Cast(type=sgl 0.0, x=w432) -> ()  [unwired: 1 out]
            n257 = Type Cast(type=sgl 0.0, x=w430) -> ()  [unwired: 1 out]
            n258 = Type Cast(type=sgl 0.0, x=w428) -> ()  [unwired: 1 out]
            n259 = Type Cast(type=sgl 0.0, x=w426) -> ()  [unwired: 1 out]
            n260 = Type Cast(type=u32 0, x=w440) -> ()  [unwired: 1 out]
          }
        }
      }
      frame "ÿZ\b\u0000H\u0000" {
        w478 = 72 ("x")
        # "EKF_NAV 0x08"
        n261 = call "SBG_Ellipse_check_length_n_end (SubVI).vi"("x"=w478, "input String"=w477) -> ("is data ok?"=w475:bool)  [unwired: 7 in, 2 out]
        n262 = case shown="True" w475 {
          tunnel: w477 -> [w479 w560]
          tunnel: [w479 w510] -> w476
          tunnel: w478 -> [_ w543]
          frame False {
          }
          frame True {
            w511 = 6 ("length (len. of substring)")
            # "Status"
            # "altitude_acc"
            # "longitude_acc"
            # "latitude_acc"
            # "undulation"
            # "altitude"
            # "longitude"
            # "latitude"
            # "velo_d_acc"
            # "Velo_E_acc"
            # "Velo_n_acc"
            # "Velocity_D"
            # "Velocity_E"
            # "Velocity_N"
            # "Time Stamp"
            n263 = Replace Substring(2:w543, 3:w511, 5:w560) -> (0:w528:string, 1:w512:string)  [unwired: 1 in]
            n264 = Replace Substring(2:w511, 5:w512) -> (1:w510:string)  [unwired: 2 in, 1 out]
            n265 = String Subset(string=w528, offset (0)=56 ("length (len. of substring)"), length (rest)=4 ("length (len. of substring)")) -> (substring=w487:string)
            n266 = String Subset(string=w528, offset (0)=52 ("length (len. of substring)"), length (rest)=4 ("length (len. of substring)")) -> (substring=w489:string)
            n267 = String Subset(string=w528, offset (0)=60 ("length (len. of substring)"), length (rest)=4 ("length (len. of substring)")) -> (substring=w485:string)
            n268 = String Subset(string=w528, offset (0)=68 ("length (len. of substring)"), length (rest)=4 ("length (len. of substring)")) -> (substring=w481:string)
            n269 = String Subset(string=w528, offset (0)=8 ("length (len. of substring)"), length (rest)=4 ("length (len. of substring)")) -> (substring=w505:string)
            n270 = String Subset(string=w528, offset (0)=64 ("length (len. of substring)"), length (rest)=4 ("length (len. of substring)")) -> (substring=w483:string)
            n271 = String Subset(string=w528, offset (0)=4 ("length (len. of substring)"), length (rest)=4 ("length (len. of substring)")) -> (substring=w507:string)
            n272 = String Subset(string=w528, offset (0)=36 ("length (len. of substring)"), length (rest)=8 ("length (len. of substring)")) -> (substring=w493:string)
            n273 = String Subset(string=w528, offset (0)=44 ("length (len. of substring)"), length (rest)=8 ("length (len. of substring)")) -> (substring=w491:string)
            n274 = String Subset(string=w528, offset (0)=12 ("length (len. of substring)"), length (rest)=4 ("length (len. of substring)")) -> (substring=w503:string)
            n275 = String Subset(string=w528, offset (0)=20 ("length (len. of substring)"), length (rest)=4 ("length (len. of substring)")) -> (substring=w499:string)
            n276 = String Subset(string=w528, offset (0)=28 ("length (len. of substring)"), length (rest)=8 ("length (len. of substring)")) -> (substring=w495:string)
            n277 = String Subset(string=w528, offset (0)=16 ("length (len. of substring)"), length (rest)=4 ("length (len. of substring)")) -> (substring=w501:string)
            n278 = String Subset(string=w528, offset (0)=0 ("length (len. of substring)"), length (rest)=4 ("length (len. of substring)")) -> (substring=w509:string)
            n279 = String Subset(string=w528, offset (0)=24 ("length (len. of substring)"), length (rest)=4 ("length (len. of substring)")) -> (substring=w497:string)
            n280 = call "SBG_Ellipse_convert_to_little_endian (SubVI).vi"("string"=w493) -> ("String"=w492:string)  [unwired: 4 in]
            n281 = call "SBG_Ellipse_convert_to_little_endian (SubVI).vi"("string"=w491) -> ("String"=w490:string)  [unwired: 4 in]
            n282 = call "SBG_Ellipse_convert_to_little_endian (SubVI).vi"("string"=w489) -> ("String"=w488:string)  [unwired: 4 in]
            n283 = call "SBG_Ellipse_convert_to_little_endian (SubVI).vi"("string"=w487) -> ("String"=w486:string)  [unwired: 4 in]
            n284 = call "SBG_Ellipse_convert_to_little_endian (SubVI).vi"("string"=w485) -> ("String"=w484:string)  [unwired: 4 in]
            n285 = call "SBG_Ellipse_convert_to_little_endian (SubVI).vi"("string"=w483) -> ("String"=w482:string)  [unwired: 4 in]
            n286 = call "SBG_Ellipse_convert_to_little_endian (SubVI).vi"("string"=w481) -> ("String"=w480:string)  [unwired: 4 in]
            n287 = call "SBG_Ellipse_convert_to_little_endian (SubVI).vi"("string"=w509) -> ("String"=w508:string)  [unwired: 4 in]
            n288 = call "SBG_Ellipse_convert_to_little_endian (SubVI).vi"("string"=w507) -> ("String"=w506:string)  [unwired: 4 in]
            n289 = call "SBG_Ellipse_convert_to_little_endian (SubVI).vi"("string"=w505) -> ("String"=w504:string)  [unwired: 4 in]
            n290 = call "SBG_Ellipse_convert_to_little_endian (SubVI).vi"("string"=w503) -> ("String"=w502:string)  [unwired: 4 in]
            n291 = call "SBG_Ellipse_convert_to_little_endian (SubVI).vi"("string"=w501) -> ("String"=w500:string)  [unwired: 4 in]
            n292 = call "SBG_Ellipse_convert_to_little_endian (SubVI).vi"("string"=w499) -> ("String"=w498:string)  [unwired: 4 in]
            n293 = call "SBG_Ellipse_convert_to_little_endian (SubVI).vi"("string"=w497) -> ("String"=w496:string)  [unwired: 4 in]
            n294 = call "SBG_Ellipse_convert_to_little_endian (SubVI).vi"("string"=w495) -> ("String"=w494:string)  [unwired: 4 in]
            n295 = Type Cast(type=u32 0, x=w480) -> ()  [unwired: 1 out]
            n296 = Type Cast(type=sgl 0.0, x=w482) -> ()  [unwired: 1 out]
            n297 = Type Cast(type=sgl 0.0, x=w506) -> ()  [unwired: 1 out]
            n298 = Type Cast(type=sgl 0.0, x=w504) -> ()  [unwired: 1 out]
            n299 = Type Cast(type=sgl 0.0, x=w502) -> ()  [unwired: 1 out]
            n300 = Type Cast(type=sgl 0.0, x=w500) -> ()  [unwired: 1 out]
            n301 = Type Cast(type=sgl 0.0, x=w498) -> ()  [unwired: 1 out]
            n302 = Type Cast(type=sgl 0.0, x=w496) -> ()  [unwired: 1 out]
            n303 = Type Cast(type=0.0, x=w494) -> ()  [unwired: 1 out]
            n304 = Type Cast(type=u32 0, x=w508) -> ()  [unwired: 1 out]
            n305 = Type Cast(type=0.0, x=w492) -> ()  [unwired: 1 out]
            n306 = Type Cast(type=0.0, x=w490) -> ()  [unwired: 1 out]
            n307 = Type Cast(type=sgl 0.0, x=w488) -> ()  [unwired: 1 out]
            n308 = Type Cast(type=sgl 0.0, x=w486) -> ()  [unwired: 1 out]
            n309 = Type Cast(type=sgl 0.0, x=w484) -> ()  [unwired: 1 out]
          }
        }
      }
      frame "ÿZ\t\u0000.\u0000" {
        w564 = 46 ("x")
        # "SHIP_MOTION 0x09"
        n310 = call "SBG_Ellipse_check_length_n_end (SubVI).vi"("x"=w564, "input String"=w563) -> ("is data ok?"=w562:bool)  [unwired: 7 in, 2 out]
        n311 = case shown="True" w562 {
          tunnel: w563 -> [w565 w631]
          tunnel: [w565 w600] -> w561
          tunnel: w564 -> [_ w614]
          frame False {
          }
          frame True {
            w601 = 6 ("length (len. of substring)")
            # "HEAVE_STATUS"
            # "VEL_Z"
            # "VEL_Y"
            # "VEL_X"
            # "ACC_Z"
            # "ACC_Y"
            # "ACC_X"
            # "HEAVE"
            # "SWAY"
            # "SURGE"
            # "HEAVE PERIOD"
            # "Time Stamp"
            n312 = Replace Substring(2:w614, 3:w601, 5:w631) -> (0:w566:string, 1:w602:string)  [unwired: 1 in]
            n313 = Replace Substring(2:w601, 5:w602) -> (1:w600:string)  [unwired: 2 in, 1 out]
            n314 = String Subset(string=w566, offset (0)=32 ("length (len. of substring)"), length (rest)=4 ("length (len. of substring)")) -> (substring=w581:string)
            n315 = String Subset(string=w566, offset (0)=8 ("length (len. of substring)"), length (rest)=4 ("length (len. of substring)")) -> (substring=w595:string)
            n316 = String Subset(string=w566, offset (0)=4 ("length (len. of substring)"), length (rest)=4 ("length (len. of substring)")) -> (substring=w597:string)
            n317 = String Subset(string=w566, offset (0)=32 ("length (len. of substring)"), length (rest)=4 ("length (len. of substring)")) -> (substring=w582:string)
            n318 = String Subset(string=w566, offset (0)=28 ("length (len. of substring)"), length (rest)=4 ("length (len. of substring)")) -> (substring=w578:string)
            n319 = String Subset(string=w566, offset (0)=12 ("length (len. of substring)"), length (rest)=4 ("length (len. of substring)")) -> (substring=w593:string)
            n320 = String Subset(string=w566, offset (0)=20 ("length (len. of substring)"), length (rest)=4 ("length (len. of substring)")) -> (substring=w589:string)
            n321 = String Subset(string=w566, offset (0)=28 ("length (len. of substring)"), length (rest)=4 ("length (len. of substring)")) -> (substring=w585:string)
            n322 = String Subset(string=w566, offset (0)=24 ("length (len. of substring)"), length (rest)=4 ("length (len. of substring)")) -> (substring=w576:string)
            n323 = String Subset(string=w566, offset (0)=16 ("length (len. of substring)"), length (rest)=4 ("length (len. of substring)")) -> (substring=w591:string)
            n324 = String Subset(string=w566, offset (0)=0 ("length (len. of substring)"), length (rest)=4 ("length (len. of substring)")) -> (substring=w599:string)
            n325 = String Subset(string=w566, offset (0)=24 ("length (len. of substring)"), length (rest)=4 ("length (len. of substring)")) -> (substring=w587:string)
            n326 = call "SBG_Ellipse_convert_to_little_endian (SubVI).vi"("string"=w576) -> ("String"=w577:string)  [unwired: 4 in]
            n327 = call "SBG_Ellipse_convert_to_little_endian (SubVI).vi"("string"=w578) -> ("String"=w579:string)  [unwired: 4 in]
            n328 = call "SBG_Ellipse_convert_to_little_endian (SubVI).vi"("string"=w581) -> ("String"=w580:string)  [unwired: 4 in]
            n329 = call "SBG_Ellipse_convert_to_little_endian (SubVI).vi"("string"=w599) -> ("String"=w598:string)  [unwired: 4 in]
            n330 = call "SBG_Ellipse_convert_to_little_endian (SubVI).vi"("string"=w597) -> ("String"=w596:string)  [unwired: 4 in]
            n331 = call "SBG_Ellipse_convert_to_little_endian (SubVI).vi"("string"=w595) -> ("String"=w594:string)  [unwired: 4 in]
            n332 = call "SBG_Ellipse_convert_to_little_endian (SubVI).vi"("string"=w593) -> ("String"=w592:string)  [unwired: 4 in]
            n333 = call "SBG_Ellipse_convert_to_little_endian (SubVI).vi"("string"=w591) -> ("String"=w590:string)  [unwired: 4 in]
            n334 = call "SBG_Ellipse_convert_to_little_endian (SubVI).vi"("string"=w589) -> ("String"=w588:string)  [unwired: 4 in]
            n335 = call "SBG_Ellipse_convert_to_little_endian (SubVI).vi"("string"=w587) -> ("String"=w586:string)  [unwired: 4 in]
            n336 = call "SBG_Ellipse_convert_to_little_endian (SubVI).vi"("string"=w585) -> ("String"=w584:string)  [unwired: 4 in]
            n337 = call "SBG_Ellipse_convert_to_little_endian (SubVI).vi"("string"=w582) -> ("String"=w583:string)  [unwired: 4 in]
            n338 = Type Cast(type=u16 0, x=w580) -> ()  [unwired: 1 out]
            n339 = Type Cast(type=sgl 0.0, x=w577) -> ()  [unwired: 1 out]
            n340 = Type Cast(type=sgl 0.0, x=w579) -> ()  [unwired: 1 out]
            n341 = Type Cast(type=sgl 0.0, x=w583) -> ()  [unwired: 1 out]
            n342 = Type Cast(type=sgl 0.0, x=w596) -> ()  [unwired: 1 out]
            n343 = Type Cast(type=sgl 0.0, x=w594) -> ()  [unwired: 1 out]
            n344 = Type Cast(type=sgl 0.0, x=w592) -> ()  [unwired: 1 out]
            n345 = Type Cast(type=sgl 0.0, x=w590) -> ()  [unwired: 1 out]
            n346 = Type Cast(type=sgl 0.0, x=w588) -> ()  [unwired: 1 out]
            n347 = Type Cast(type=sgl 0.0, x=w586) -> ()  [unwired: 1 out]
            n348 = Type Cast(type=sgl 0.0, x=w584) -> ()  [unwired: 1 out]
            n349 = Type Cast(type=u32 0, x=w598) -> ()  [unwired: 1 out]
          }
        }
      }
      frame "ÿZ\r\u0000,\u0000" {
        w635 = 44 ("x")
        # "GPS1_Vel 0x0D"
        n350 = call "SBG_Ellipse_check_length_n_end (SubVI).vi"("x"=w635, "input String"=w632) -> ("is data ok?"=w633:bool)  [unwired: 7 in, 2 out]
        n351 = case shown="True" w633 {
          tunnel: w632 -> [w636 w697]
          tunnel: [w636 w659] -> w634
          tunnel: w635 -> [_ w680]
          frame False {
          }
          frame True {
            w660 = 6 ("length (len. of substring)")
            # "course_acc"
            # "course"
            # "vel_acc_d"
            # "vel_acc_e"
            # "vel_acc_n"
            # "Vel_d"
            # "Vel_e"
            # "Vel_n"
            # "GPS_tow"
            # "GPS_Vel_status"
            # "Time Stamp"
            n352 = Replace Substring(2:w680, 3:w660, 5:w697) -> (0:w673:string, 1:w661:string)  [unwired: 1 in]
            n353 = Replace Substring(2:w660, 5:w661) -> (1:w659:string)  [unwired: 2 in, 1 out]
            n354 = String Subset(string=w673, offset (0)=40 ("length (len. of substring)"), length (rest)=4 ("length (len. of substring)")) -> (substring=w638:string)
            n355 = String Subset(string=w673, offset (0)=8 ("length (len. of substring)"), length (rest)=4 ("length (len. of substring)")) -> (substring=w654:string)
            n356 = String Subset(string=w673, offset (0)=36 ("length (len. of substring)"), length (rest)=4 ("length (len. of substring)")) -> (substring=w640:string)
            n357 = String Subset(string=w673, offset (0)=4 ("length (len. of substring)"), length (rest)=4 ("length (len. of substring)")) -> (substring=w656:string)
            n358 = String Subset(string=w673, offset (0)=32 ("length (len. of substring)"), length (rest)=4 ("length (len. of substring)")) -> (substring=w641:string)
            n359 = String Subset(string=w673, offset (0)=12 ("length (len. of substring)"), length (rest)=4 ("length (len. of substring)")) -> (substring=w652:string)
            n360 = String Subset(string=w673, offset (0)=20 ("length (len. of substring)"), length (rest)=4 ("length (len. of substring)")) -> (substring=w648:string)
            n361 = String Subset(string=w673, offset (0)=28 ("length (len. of substring)"), length (rest)=4 ("length (len. of substring)")) -> (substring=w644:string)
            n362 = String Subset(string=w673, offset (0)=16 ("length (len. of substring)"), length (rest)=4 ("length (len. of substring)")) -> (substring=w650:string)
            n363 = String Subset(string=w673, offset (0)=0 ("length (len. of substring)"), length (rest)=4 ("length (len. of substring)")) -> (substring=w658:string)
            n364 = String Subset(string=w673, offset (0)=24 ("length (len. of substring)"), length (rest)=4 ("length (len. of substring)")) -> (substring=w646:string)
            n365 = call "SBG_Ellipse_convert_to_little_endian (SubVI).vi"("string"=w641) -> ("String"=w642:string)  [unwired: 4 in]
            n366 = call "SBG_Ellipse_convert_to_little_endian (SubVI).vi"("string"=w640) -> ("String"=w639:string)  [unwired: 4 in]
            n367 = call "SBG_Ellipse_convert_to_little_endian (SubVI).vi"("string"=w638) -> ("String"=w637:string)  [unwired: 4 in]
            n368 = call "SBG_Ellipse_convert_to_little_endian (SubVI).vi"("string"=w658) -> ("String"=w657:string)  [unwired: 4 in]
            n369 = call "SBG_Ellipse_convert_to_little_endian (SubVI).vi"("string"=w656) -> ("String"=w655:string)  [unwired: 4 in]
            n370 = call "SBG_Ellipse_convert_to_little_endian (SubVI).vi"("string"=w654) -> ("String"=w653:string)  [unwired: 4 in]
            n371 = call "SBG_Ellipse_convert_to_little_endian (SubVI).vi"("string"=w652) -> ("String"=w651:string)  [unwired: 4 in]
            n372 = call "SBG_Ellipse_convert_to_little_endian (SubVI).vi"("string"=w650) -> ("String"=w649:string)  [unwired: 4 in]
            n373 = call "SBG_Ellipse_convert_to_little_endian (SubVI).vi"("string"=w648) -> ("String"=w647:string)  [unwired: 4 in]
            n374 = call "SBG_Ellipse_convert_to_little_endian (SubVI).vi"("string"=w646) -> ("String"=w645:string)  [unwired: 4 in]
            n375 = call "SBG_Ellipse_convert_to_little_endian (SubVI).vi"("string"=w644) -> ("String"=w643:string)  [unwired: 4 in]
            n376 = Type Cast(type=u32 0, x=w657) -> ()  [unwired: 1 out]
            n377 = Type Cast(type=u32 0, x=w655) -> ()  [unwired: 1 out]
            n378 = Type Cast(type=u32 0, x=w653) -> ()  [unwired: 1 out]
            n379 = Type Cast(type=sgl 0.0, x=w643) -> ()  [unwired: 1 out]
            n380 = Type Cast(type=sgl 0.0, x=w642) -> ()  [unwired: 1 out]
            n381 = Type Cast(type=sgl 0.0, x=w639) -> ()  [unwired: 1 out]
            n382 = Type Cast(type=sgl 0.0, x=w637) -> ()  [unwired: 1 out]
            n383 = Type Cast(type=sgl 0.0, x=w651) -> ()  [unwired: 1 out]
            n384 = Type Cast(type=sgl 0.0, x=w649) -> ()  [unwired: 1 out]
            n385 = Type Cast(type=sgl 0.0, x=w647) -> ()  [unwired: 1 out]
            n386 = Type Cast(type=sgl 0.0, x=w645) -> ()  [unwired: 1 out]
          }
        }
      }
      frame "ÿZ\u000e\u00009\u0000" {
        w701 = 57 ("x")
        # "GPS1_Pos 0x0E"
        n387 = call "SBG_Ellipse_check_length_n_end (SubVI).vi"("x"=w701, "input String"=w700) -> ("is data ok?"=w698:bool)  [unwired: 7 in, 2 out]
        n388 = case shown="True" w698 {
          tunnel: w700 -> [w702 w773]
          tunnel: [w702 w731] -> w699
          tunnel: w701 -> [_ w756]
          frame False {
          }
          frame True {
            w730 = 6 ("length (len. of substring)")
            # "diff_age"
            # "base_sation_id"
            # "num_sv_used"
            # "pos_acc_alt"
            # "pos_acc_long"
            # "pos_acc_lat"
            # "undulation"
            # "altitude"
            # "long"
            # "lat"
            # "GPS_tow"
            # "GPS_pos_status"
            # "Time Stamp"
            n389 = Replace Substring(2:w756, 3:w730, 5:w773) -> (0:w745:string, 1:w729:string)  [unwired: 1 in]
            n390 = Replace Substring(2:w730, 5:w729) -> (1:w731:string)  [unwired: 2 in, 1 out]
            n391 = String Subset(string=w745, offset (0)=54 ("length (len. of substring)"), length (rest)=2 ("length (len. of substring)")) -> (substring=w706:string)
            n392 = String Subset(string=w745, offset (0)=56 ("length (len. of substring)"), length (rest)=2 ("length (len. of substring)")) -> (substring=w704:string)
            n393 = String Subset(string=w745, offset (0)=52 ("length (len. of substring)"), length (rest)=1 ("length (len. of substring)")) -> (substring=w707:string)
            n394 = String Subset(string=w745, offset (0)=8 ("length (len. of substring)"), length (rest)=4 ("length (len. of substring)")) -> (substring=w724:string)
            n395 = String Subset(string=w745, offset (0)=48 ("length (len. of substring)"), length (rest)=4 ("length (len. of substring)")) -> (substring=w710:string)
            n396 = String Subset(string=w745, offset (0)=4 ("length (len. of substring)"), length (rest)=4 ("length (len. of substring)")) -> (substring=w726:string)
            n397 = String Subset(string=w745, offset (0)=44 ("length (len. of substring)"), length (rest)=4 ("length (len. of substring)")) -> (substring=w712:string)
            n398 = String Subset(string=w745, offset (0)=12 ("length (len. of substring)"), length (rest)=8 ("length (len. of substring)")) -> (substring=w722:string)
            n399 = String Subset(string=w745, offset (0)=28 ("length (len. of substring)"), length (rest)=8 ("length (len. of substring)")) -> (substring=w718:string)
            n400 = String Subset(string=w745, offset (0)=40 ("length (len. of substring)"), length (rest)=4 ("length (len. of substring)")) -> (substring=w714:string)
            n401 = String Subset(string=w745, offset (0)=20 ("length (len. of substring)"), length (rest)=8 ("length (len. of substring)")) -> (substring=w720:string)
            n402 = String Subset(string=w745, offset (0)=0 ("length (len. of substring)"), length (rest)=4 ("length (len. of substring)")) -> (substring=w728:string)
            n403 = String Subset(string=w745, offset (0)=36 ("length (len. of substring)"), length (rest)=4 ("length (len. of substring)")) -> (substring=w716:string)
            n404 = call "SBG_Ellipse_convert_to_little_endian (SubVI).vi"("string"=w712) -> ("String"=w711:string)  [unwired: 4 in]
            n405 = call "SBG_Ellipse_convert_to_little_endian (SubVI).vi"("string"=w710) -> ("String"=w709:string)  [unwired: 4 in]
            n406 = call "SBG_Ellipse_convert_to_little_endian (SubVI).vi"("string"=w707) -> ("String"=w708:string)  [unwired: 4 in]
            n407 = call "SBG_Ellipse_convert_to_little_endian (SubVI).vi"("string"=w706) -> ("String"=w705:string)  [unwired: 4 in]
            n408 = call "SBG_Ellipse_convert_to_little_endian (SubVI).vi"("string"=w704) -> ("String"=w703:string)  [unwired: 4 in]
            n409 = call "SBG_Ellipse_convert_to_little_endian (SubVI).vi"("string"=w728) -> ("String"=w727:string)  [unwired: 4 in]
            n410 = call "SBG_Ellipse_convert_to_little_endian (SubVI).vi"("string"=w726) -> ("String"=w725:string)  [unwired: 4 in]
            n411 = call "SBG_Ellipse_convert_to_little_endian (SubVI).vi"("string"=w724) -> ("String"=w723:string)  [unwired: 4 in]
            n412 = call "SBG_Ellipse_convert_to_little_endian (SubVI).vi"("string"=w722) -> ("String"=w721:string)  [unwired: 4 in]
            n413 = call "SBG_Ellipse_convert_to_little_endian (SubVI).vi"("string"=w720) -> ("String"=w719:string)  [unwired: 4 in]
            n414 = call "SBG_Ellipse_convert_to_little_endian (SubVI).vi"("string"=w718) -> ("String"=w717:string)  [unwired: 4 in]
            n415 = call "SBG_Ellipse_convert_to_little_endian (SubVI).vi"("string"=w716) -> ("String"=w715:string)  [unwired: 4 in]
            n416 = call "SBG_Ellipse_convert_to_little_endian (SubVI).vi"("string"=w714) -> ("String"=w713:string)  [unwired: 4 in]
            n417 = Type Cast(type=u32 0, x=w727) -> ()  [unwired: 1 out]
            n418 = Type Cast(type=u32 0, x=w725) -> ()  [unwired: 1 out]
            n419 = Type Cast(type=u32 0, x=w723) -> ()  [unwired: 1 out]
            n420 = Type Cast(type=0.0, x=w721) -> ()  [unwired: 1 out]
            n421 = Type Cast(type=0.0, x=w719) -> ()  [unwired: 1 out]
            n422 = Type Cast(type=0.0, x=w717) -> ()  [unwired: 1 out]
            n423 = Type Cast(type=sgl 0.0, x=w715) -> ()  [unwired: 1 out]
            n424 = Type Cast(type=sgl 0.0, x=w713) -> ()  [unwired: 1 out]
            n425 = Type Cast(type=sgl 0.0, x=w711) -> ()  [unwired: 1 out]
            n426 = Type Cast(type=sgl 0.0, x=w709) -> ()  [unwired: 1 out]
            n427 = Type Cast(type=u8 0, x=w708) -> ()  [unwired: 1 out]
            n428 = Type Cast(type=u16 0, x=w705) -> ()  [unwired: 1 out]
            n429 = Type Cast(type=u16 0, x=w703) -> ()  [unwired: 1 out]
          }
        }
      }
      frame "ÿZ\u000f\u0000\u001a\u0000" {
        w777 = 26 ("x")
        # "GPS1_HDT 0x0F"
        n430 = call "SBG_Ellipse_check_length_n_end (SubVI).vi"("x"=w777, "input String"=w776) -> ("is data ok?"=w774:bool)  [unwired: 7 in, 2 out]
        n431 = case shown="True" w774 {
          tunnel: w776 -> [w778 w819]
          tunnel: [w778 w795] -> w775
          tunnel: w777 -> [_ w804]
          frame False {
          }
          frame True {
            w793 = 6 ("length (len. of substring)")
            # "GPS PITCH ACC"
            # "GPS PITCH"
            # "GPS HEADING ACC"
            # "GPS TRUE HEADING"
            # "GPS_tow"
            # "GPS HDT STATUS"
            # "Time Stamp"
            n432 = Replace Substring(2:w804, 3:w793, 5:w819) -> (0:w803:string, 1:w794:string)  [unwired: 1 in]
            n433 = Replace Substring(2:w793, 5:w794) -> (1:w795:string)  [unwired: 2 in, 1 out]
            n434 = String Subset(string=w803, offset (0)=6 ("length (len. of substring)"), length (rest)=4 ("length (len. of substring)")) -> (substring=w780:string)
            n435 = String Subset(string=w803, offset (0)=4 ("length (len. of substring)"), length (rest)=2 ("length (len. of substring)")) -> (substring=w790:string)
            n436 = String Subset(string=w803, offset (0)=10 ("length (len. of substring)"), length (rest)=4 ("length (len. of substring)")) -> (substring=w782:string)
            n437 = String Subset(string=w803, offset (0)=18 ("length (len. of substring)"), length (rest)=4 ("length (len. of substring)")) -> (substring=w786:string)
            n438 = String Subset(string=w803, offset (0)=14 ("length (len. of substring)"), length (rest)=4 ("length (len. of substring)")) -> (substring=w784:string)
            n439 = String Subset(string=w803, offset (0)=0 ("length (len. of substring)"), length (rest)=4 ("length (len. of substring)")) -> (substring=w792:string)
            n440 = String Subset(string=w803, offset (0)=22 ("length (len. of substring)"), length (rest)=4 ("length (len. of substring)")) -> (substring=w788:string)
            n441 = call "SBG_Ellipse_convert_to_little_endian (SubVI).vi"("string"=w792) -> ("String"=w791:string)  [unwired: 4 in]
            n442 = call "SBG_Ellipse_convert_to_little_endian (SubVI).vi"("string"=w790) -> ("String"=w789:string)  [unwired: 4 in]
            n443 = call "SBG_Ellipse_convert_to_little_endian (SubVI).vi"("string"=w780) -> ("String"=w779:string)  [unwired: 4 in]
            n444 = call "SBG_Ellipse_convert_to_little_endian (SubVI).vi"("string"=w782) -> ("String"=w781:string)  [unwired: 4 in]
            n445 = call "SBG_Ellipse_convert_to_little_endian (SubVI).vi"("string"=w784) -> ("String"=w783:string)  [unwired: 4 in]
            n446 = call "SBG_Ellipse_convert_to_little_endian (SubVI).vi"("string"=w786) -> ("String"=w785:string)  [unwired: 4 in]
            n447 = call "SBG_Ellipse_convert_to_little_endian (SubVI).vi"("string"=w788) -> ("String"=w787:string)  [unwired: 4 in]
            n448 = Type Cast(type=u32 0, x=w791) -> ()  [unwired: 1 out]
            n449 = Type Cast(type=u16 0, x=w789) -> ()  [unwired: 1 out]
            n450 = Type Cast(type=u32 0, x=w779) -> ()  [unwired: 1 out]
            n451 = Type Cast(type=sgl 0.0, x=w781) -> ()  [unwired: 1 out]
            n452 = Type Cast(type=sgl 0.0, x=w783) -> ()  [unwired: 1 out]
            n453 = Type Cast(type=sgl 0.0, x=w785) -> ()  [unwired: 1 out]
            n454 = Type Cast(type=sgl 0.0, x=w787) -> ()  [unwired: 1 out]
          }
        }
      }
      frame "ÿZ\u0013\u0000\n\u0000" {
        w823 = 10 ("x")
        # "ODO_VEL 0x13"
        n455 = call "SBG_Ellipse_check_length_n_end (SubVI).vi"("x"=w823, "input String"=w822) -> ("is data ok?"=w820:bool)  [unwired: 7 in, 2 out]
        n456 = case shown="True" w820 {
          tunnel: w822 -> [w824 w846]
          tunnel: [w824 w832] -> w821
          tunnel: w823 -> [_ w839]
          frame False {
          }
          frame True {
            w833 = 6 ("length (len. of substring)")
            # "ODO_VEL"
            # "ODO_STATUS"
            # "Time Stamp"
            n457 = Replace Substring(2:w839, 3:w833, 5:w846) -> (0:w838:string, 1:w834:string)  [unwired: 1 in]
            n458 = Replace Substring(2:w833, 5:w834) -> (1:w832:string)  [unwired: 2 in, 1 out]
            n459 = String Subset(string=w838, offset (0)=6 ("length (len. of substring)"), length (rest)=4 ("length (len. of substring)")) -> (substring=w827:string)
            n460 = String Subset(string=w838, offset (0)=4 ("length (len. of substring)"), length (rest)=2 ("length (len. of substring)")) -> (substring=w829:string)
            n461 = String Subset(string=w838, offset (0)=0 ("length (len. of substring)"), length (rest)=4 ("length (len. of substring)")) -> (substring=w831:string)
            n462 = call "SBG_Ellipse_convert_to_little_endian (SubVI).vi"("string"=w831) -> ("String"=w830:string)  [unwired: 4 in]
            n463 = call "SBG_Ellipse_convert_to_little_endian (SubVI).vi"("string"=w829) -> ("String"=w828:string)  [unwired: 4 in]
            n464 = call "SBG_Ellipse_convert_to_little_endian (SubVI).vi"("string"=w827) -> ("String"=w826:string)  [unwired: 4 in]
            n465 = Type Cast(type=u16 0, x=w828) -> ()  [unwired: 1 out]
            n466 = Type Cast(type=sgl 0.0, x=w826) -> (*(type *) &x=w825:sgl)
            n467 = Type Cast(type=u32 0, x=w830) -> ()  [unwired: 1 out]
            n468 = To Double Precision Float(number=w825) -> ()  [unwired: 1 out]
          }
        }
      }
      frame "ÿZ\u0018\u0000\u000e\u0000" {
        w850 = 14 ("x")
        # "EVENT_A 0x18"
        # "EVENT_A 0x18"
        n469 = call "SBG_Ellipse_check_length_n_end (SubVI).vi"("x"=w850, "input String"=w849) -> ("is data ok?"=w847:bool)  [unwired: 7 in, 2 out]
        n470 = case shown="True" w847 {
          tunnel: w849 -> [w851 w887]
          tunnel: [w851 w865] -> w848
          tunnel: w850 -> [_ w874]
          frame False {
          }
          frame True {
            w864 = 6 ("length (len. of substring)")
            # "TIME OFFSET_3"
            # "TIME OFFSET_2"
            # "TIME OFFSET_1"
            # "TIME OFFSET_0"
            # "EVENT STATUS"
            # "Time Stamp"
            n471 = Replace Substring(2:w874, 3:w864, 5:w887) -> (0:w873:string, 1:w866:string)  [unwired: 1 in]
            n472 = Replace Substring(2:w864, 5:w866) -> (1:w865:string)  [unwired: 2 in, 1 out]
            n473 = String Subset(string=w873, offset (0)=6 ("length (len. of substring)"), length (rest)=2 ("length (len. of substring)")) -> (substring=w859:string)
            n474 = String Subset(string=w873, offset (0)=4 ("length (len. of substring)"), length (rest)=2 ("length (len. of substring)")) -> (substring=w861:string)
            n475 = String Subset(string=w873, offset (0)=8 ("length (len. of substring)"), length (rest)=2 ("length (len. of substring)")) -> (substring=w857:string)
            n476 = String Subset(string=w873, offset (0)=12 ("length (len. of substring)"), length (rest)=2 ("length (len. of substring)")) -> (substring=w853:string)
            n477 = String Subset(string=w873, offset (0)=10 ("length (len. of substring)"), length (rest)=2 ("length (len. of substring)")) -> (substring=w855:string)
            n478 = String Subset(string=w873, offset (0)=0 ("length (len. of substring)"), length (rest)=4 ("length (len. of substring)")) -> (substring=w863:string)
            n479 = call "SBG_Ellipse_convert_to_little_endian (SubVI).vi"("string"=w863) -> ("String"=w862:string)  [unwired: 4 in]
            n480 = call "SBG_Ellipse_convert_to_little_endian (SubVI).vi"("string"=w861) -> ("String"=w860:string)  [unwired: 4 in]
            n481 = call "SBG_Ellipse_convert_to_little_endian (SubVI).vi"("string"=w859) -> ("String"=w858:string)  [unwired: 4 in]
            n482 = call "SBG_Ellipse_convert_to_little_endian (SubVI).vi"("string"=w857) -> ("String"=w856:string)  [unwired: 4 in]
            n483 = call "SBG_Ellipse_convert_to_little_endian (SubVI).vi"("string"=w855) -> ("String"=w854:string)  [unwired: 4 in]
            n484 = call "SBG_Ellipse_convert_to_little_endian (SubVI).vi"("string"=w853) -> ("String"=w852:string)  [unwired: 4 in]
            n485 = Type Cast(type=u32 0, x=w862) -> ()  [unwired: 1 out]
            n486 = Type Cast(type=u16 0, x=w860) -> ()  [unwired: 1 out]
            n487 = Type Cast(type=u16 0, x=w858) -> ()  [unwired: 1 out]
            n488 = Type Cast(type=u16 0, x=w856) -> ()  [unwired: 1 out]
            n489 = Type Cast(type=u16 0, x=w854) -> ()  [unwired: 1 out]
            n490 = Type Cast(type=u16 0, x=w852) -> ()  [unwired: 1 out]
          }
        }
      }
      frame "ÿZ$\u0000\u000e\u0000" {
        w891 = 14 ("x")
        # "PRESSURE 0x24"
        n491 = call "SBG_Ellipse_check_length_n_end (SubVI).vi"("x"=w891, "input String"=w890) -> ("is data ok?"=w888:bool)  [unwired: 7 in, 2 out]
        n492 = case shown="True" w888 {
          tunnel: w890 -> [w892 w922]
          tunnel: [w892 w905] -> w889
          tunnel: w891 -> [_ w913]
          frame False {
          }
          frame True {
            w906 = 6 ("length (len. of substring)")
            # "Altitude"
            # "Pressure"
            # "Pressure_status"
            # "Time Stamp"
            n493 = Replace Substring(2:w913, 3:w906, 5:w922) -> (0:w912:string, 1:w907:string)  [unwired: 1 in]
            n494 = Replace Substring(2:w906, 5:w907) -> (1:w905:string)  [unwired: 2 in, 1 out]
            n495 = String Subset(string=w912, offset (0)=6 ("length (len. of substring)"), length (rest)=4 ("length (len. of substring)")) -> (substring=w900:string)
            n496 = String Subset(string=w912, offset (0)=4 ("length (len. of substring)"), length (rest)=2 ("length (len. of substring)")) -> (substring=w902:string)
            n497 = String Subset(string=w912, offset (0)=10 ("length (len. of substring)"), length (rest)=4 ("length (len. of substring)")) -> (substring=w898:string)
            n498 = String Subset(string=w912, offset (0)=0 ("length (len. of substring)"), length (rest)=4 ("length (len. of substring)")) -> (substring=w904:string)
            n499 = call "SBG_Ellipse_convert_to_little_endian (SubVI).vi"("string"=w904) -> ("String"=w903:string)  [unwired: 4 in]
            n500 = call "SBG_Ellipse_convert_to_little_endian (SubVI).vi"("string"=w902) -> ("String"=w901:string)  [unwired: 4 in]
            n501 = call "SBG_Ellipse_convert_to_little_endian (SubVI).vi"("string"=w900) -> ("String"=w899:string)  [unwired: 4 in]
            n502 = call "SBG_Ellipse_convert_to_little_endian (SubVI).vi"("string"=w898) -> ("String"=w897:string)  [unwired: 4 in]
            n503 = Type Cast(type=u16 0, x=w901) -> ()  [unwired: 1 out]
            n504 = Type Cast(type=sgl 0.0, x=w899) -> (*(type *) &x=w896:sgl)
            n505 = Type Cast(type=sgl 0.0, x=w897) -> ()  [unwired: 1 out]
            n506 = Type Cast(type=u32 0, x=w903) -> ()  [unwired: 1 out]
            n507 = To Double Precision Float(number=w896) -> (double precision float=w893:dbl)
            n508 = shared-variable ".\\SingleProcessVariable.lvlib\\IMUData"() -> (w894:T1)  [unwired: 1 in, 1 out]
            n509 = Bundle By Name(cluster=w894, "Pressure (psia)"=w893) -> (w895:T1)
            n510 = shared-variable ".\\SingleProcessVariable.lvlib\\IMUData"(w895) -> ()  [unwired: 1 in, 1 out]
          }
        }
      }
    }
    n511 = call "SBG_Ellipse_starting_debug (SubVI).vi"("boolean from check"=w5, "result string in"=w8) -> ("result string out"=w12:string)  [unwired: 9 in]
    n512 = String Length(string=w12) -> (length=w15:i32)
    "buffer length" <- w15
    n513 = Greater Or Equal?(x=w15, y=10000) -> (x >= y?=w13:bool)
    n514 = Select(t="", s=w13, f=w12) -> (s? t:f=w10:string)
    n515 = feedback-in #1(w10) -> ()
    n516 = shared-variable ".\\SingleProcessVariable.lvlib\\GlobalStop"() -> (w9:bool)  [unwired: 1 in, 1 out]
  }
  "error out" <- w1
